vi "demo2.vi"() -> (0 "Error Out":errorcluster)   [LabVIEW 2024]
uses:
  Alarming-Actor/Source/Alarming Actor/Alarming Actor/Alarming Actor.lvclass
  Alarming-Actor/Source/Alarming Actor UI/Alarming Actor UI.lvclass
  Source/Alarming Strategy/Alarming Actor Strategy.lvclass
  Source/Interfaces/IRead Temperature/IRead Temperature.lvclass
  Source/Interfaces/IWrite Duty Cycle/IWrite Duty Cycle.lvclass
  Source/Interfaces/IReadPressure/IRead Pressure.lvclass
  Source/Interfaces/IRead Dew Point/IRead Dew Point.lvclass
  Source/Interfaces/IRead Humidity/IRead Humidity.lvclass
  Source/Interfaces/IRead H2O Concentration/IRead H2O Concentration.lvclass
  Source/Interfaces/IVirtual Instrument/IVirtual Instrument.lvclass
  Source/Instrument Manager/Instrument Manager.lvclass
  Source/Interfaces/IRunnable/IRunnable.lvclass
  Alarming-Actor/Source/Alarming Actor/Alarming Actor/Alarming Level.ctl
  Supply Control States.ctl
  fd6abf06-3d04-4345-ac09-30423c28f45e.vi
  f97e5bf6-71f0-418f-9a98-3962d6491cca.vi
  a312cea4-3cc5-4a6b-8bfd-08d3799cec9d.vi
  458dd3b6-fbb4-4b61-9531-a4b22eeaadbe.vi
  96793fb8-29df-4936-a506-fddfdbc4ff2a.vi
  Progress Bar Switch.ctl
  Stack.ctl
panel:
  out "Stack2":T1 {"Power-Setpoint" format="%d %"; "Purge Valve" scale=0.0..100.0; "Supply Valve" scale=0.0..100.0; "Switch" scale=0.0..100.0; "Voltage" format="%#.2f V"; "Current" format="%#.2f A"; "Pressure" format="%#.0f mbar"; "Thermometer" format="%#.1f °C"; "Fan" format="%d %"; "Power" format="%d W"}
  out "Stack1":T1 {"Power-Setpoint" format="%d %"; "Purge Valve" scale=0.0..100.0; "Supply Valve" scale=0.0..100.0; "Switch" scale=0.0..100.0; "Voltage" format="%#.2f V"; "Current" format="%#.2f A"; "Pressure" format="%#.0f mbar"; "Thermometer" format="%#.1f °C"; "Fan" format="%d %"; "Power" format="%d W"}
  out "Stack Temps":T3(graph) caption="Stack Temperatures °C"
  out "Stack Temperatures":T4(graph)
  in  "Stop Button":bool
  in  "Start Button":bool
  in  "Shutdown Button":bool
  out "Identifier":string
  out "Alarming Level":T5
  out "Temperature":dbl format="%.2f °C"
  out "Time Stamp t":timestamp format="%<%x %.3X>T"
  out "Pressure":dbl format="%d mbar a"
  out "Time Stamp p":timestamp format="%<%x %.3X>T"
  out "Dew Point":dbl format="%.2f °C"
  out "Time Stamp d":timestamp format="%<%x %.3X>T"
  out "Absolute Humidity":dbl format="%.1f g/m³"
  out "Time Stamp h":timestamp format="%<%x %.3X>T"
  out "H2O Concentration":dbl format="%d Vol.-%"
  out "Time Stamp c":timestamp format="%<%x %.3X>T"
  out "Main Supply":T6(graph)
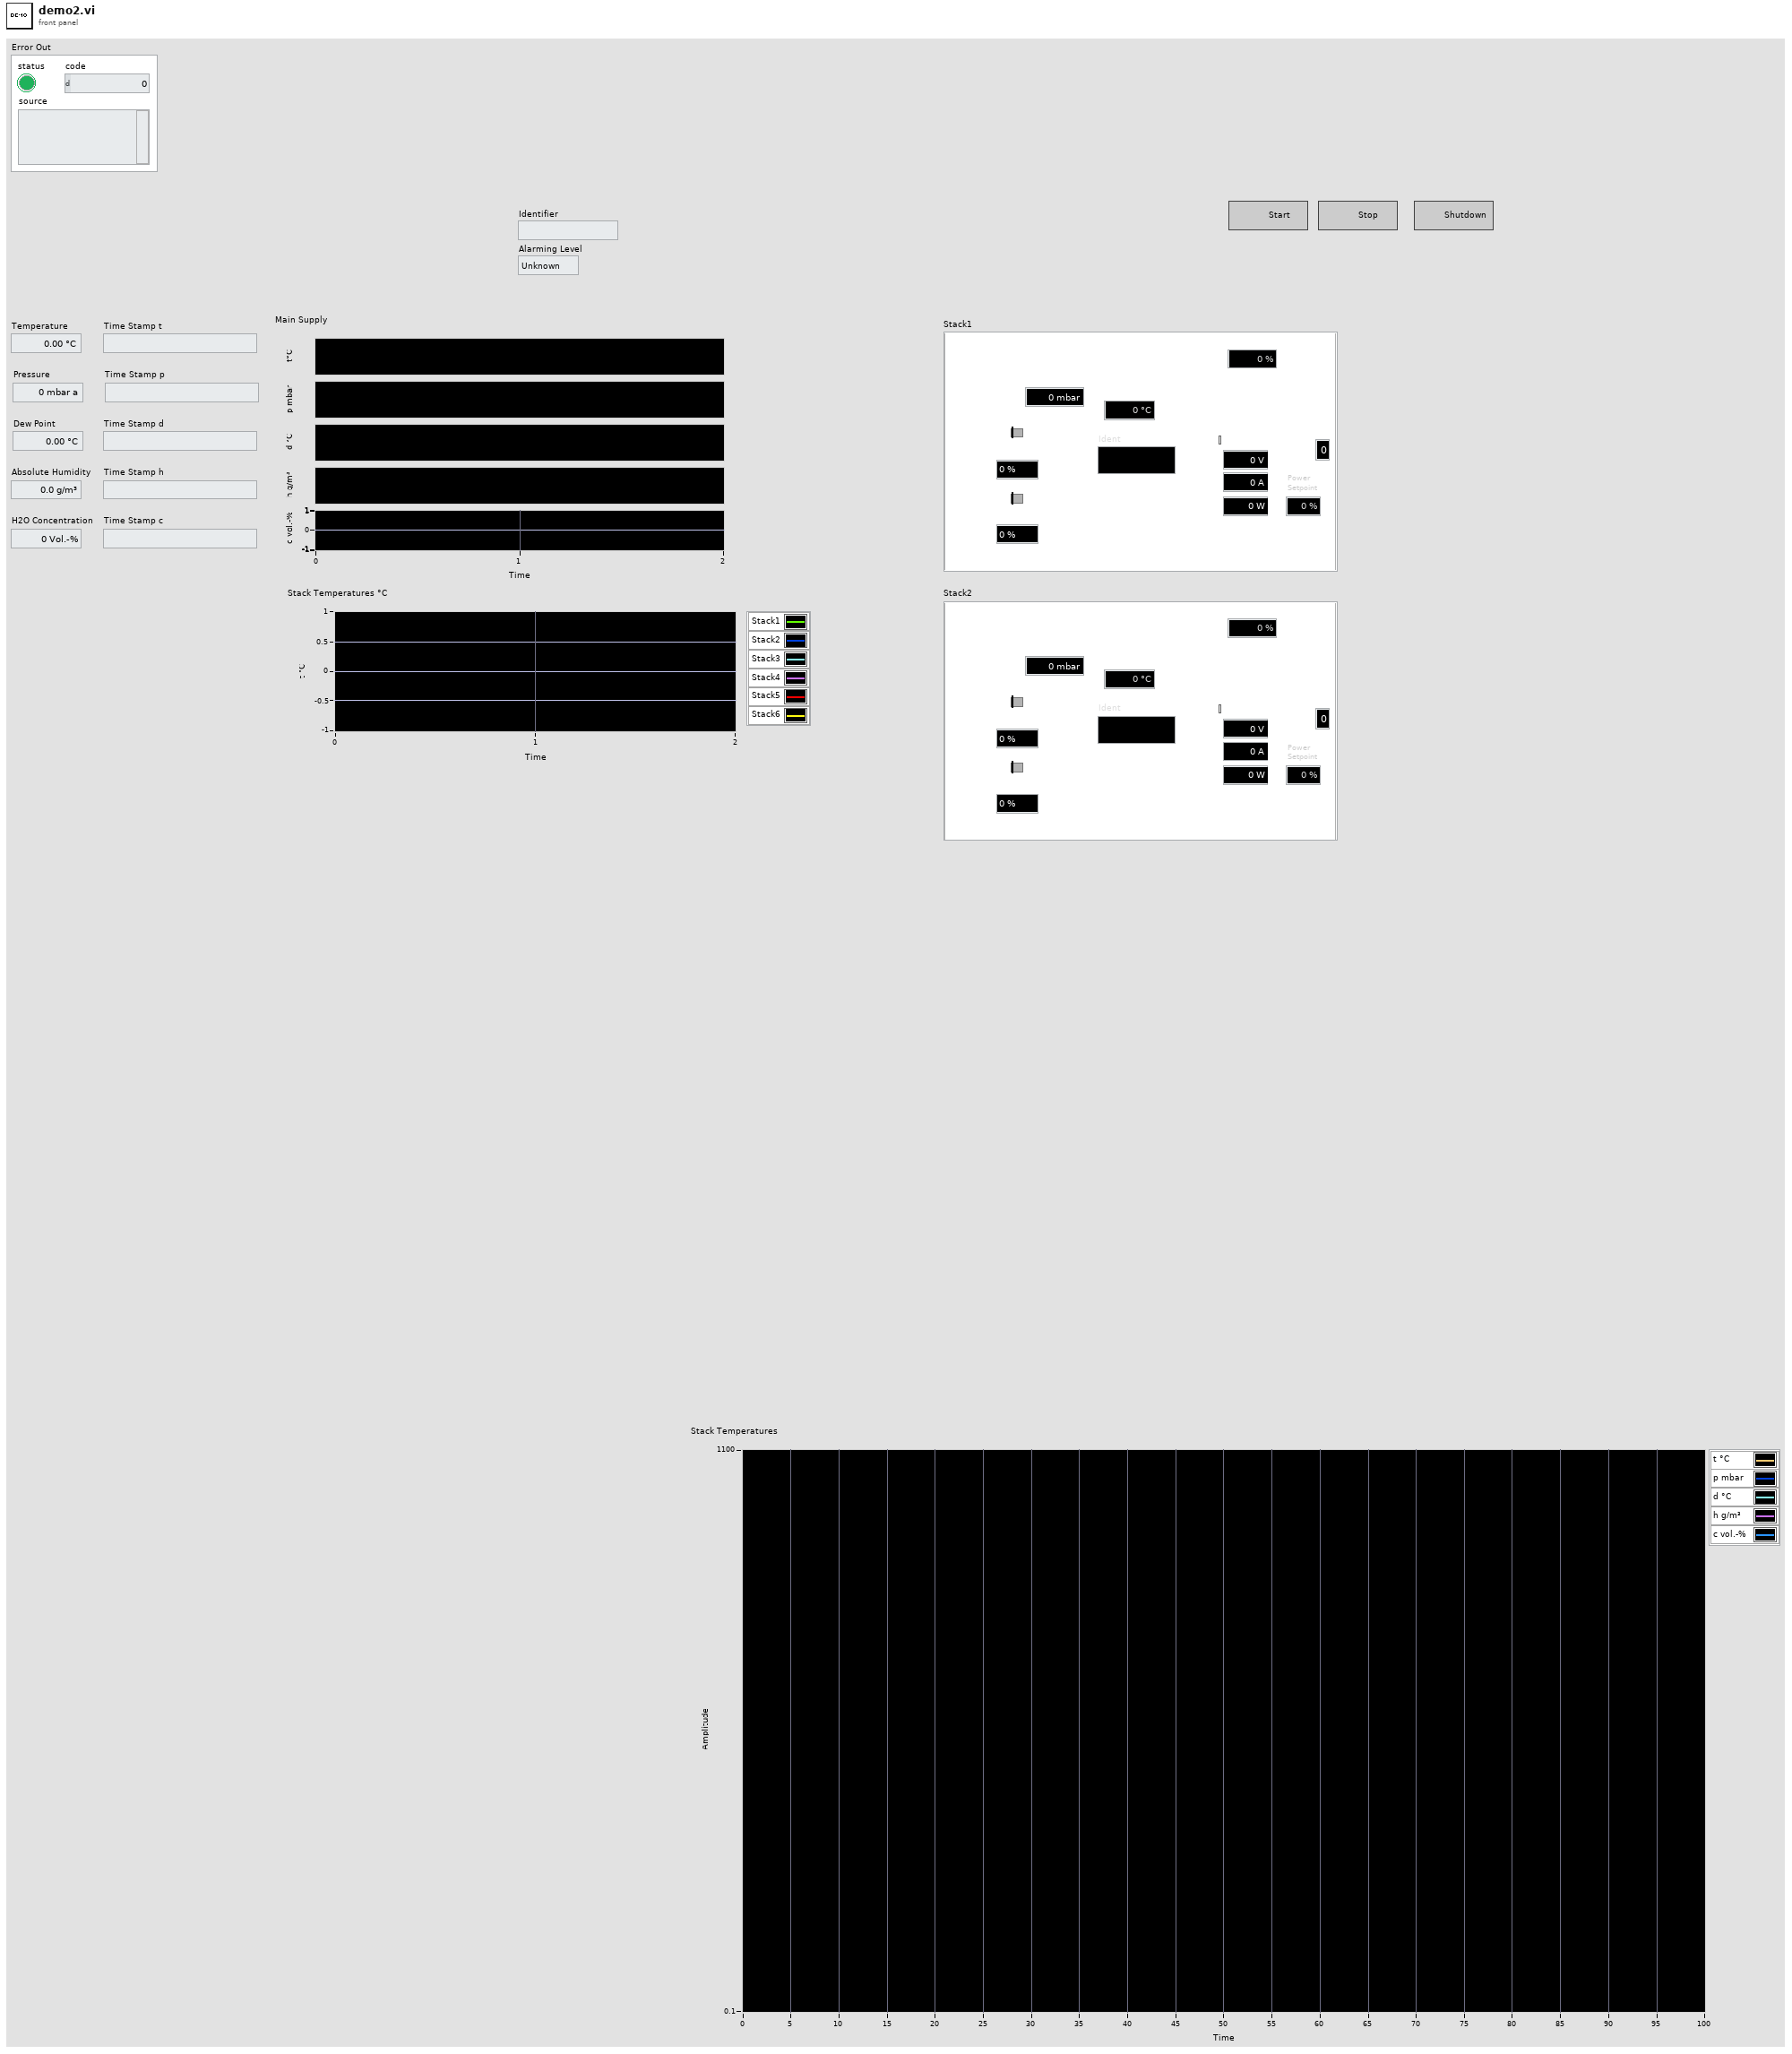
[diagram p1: front panel]
types:
  T1 = typedef "Stack.ctl" = cluster{"Ident":string, "Power":dbl, "Fan":dbl, "Thermometer":dbl, "MCU":u8, "Pressure":dbl, "Current":dbl, "Voltage":dbl, "Switch 2":bool, "Switch 3":bool, "Switch":T2, "Switch 4":bool, "Supply Valve":dbl, "Purge Valve":dbl, "Power-Setpoint":dbl}
  T2 = typedef "Progress Bar Switch.ctl" = u8
  T3 = cluster{"[0]":dbl, "[1]":dbl, "[2]":dbl, "[3]":dbl, "[4]":dbl, "[5]":dbl}
  T4 = cluster{"Temperature":dbl, "Temperature":dbl, "Temperature":dbl, "Temperature":dbl, "Temperature":dbl, "Temperature":dbl}
  T5 = typedef "Alarming Actor.lvlib/Alarming Actor.lvclass/Alarming Level.ctl" = enum16{"Unknown", "OK", "Warning", "Critical"}
  T6 = cluster{"Temperature":dbl, "Pressure":dbl, "Dew Point":dbl, "Humidity":dbl, "H2O Concentration":dbl}
  T7 = typedef "Supply Control States.ctl" = enum16{"Idle", "Run", "Shutdown"}
  T8 = cluster{"Identifier":string, "Alarming Level":T5}
  T9 = cluster{"Alarm Status Changed":refnum<user-event>}
  T10 = typedef "Rendezvous RefNum" = refnum<k1>
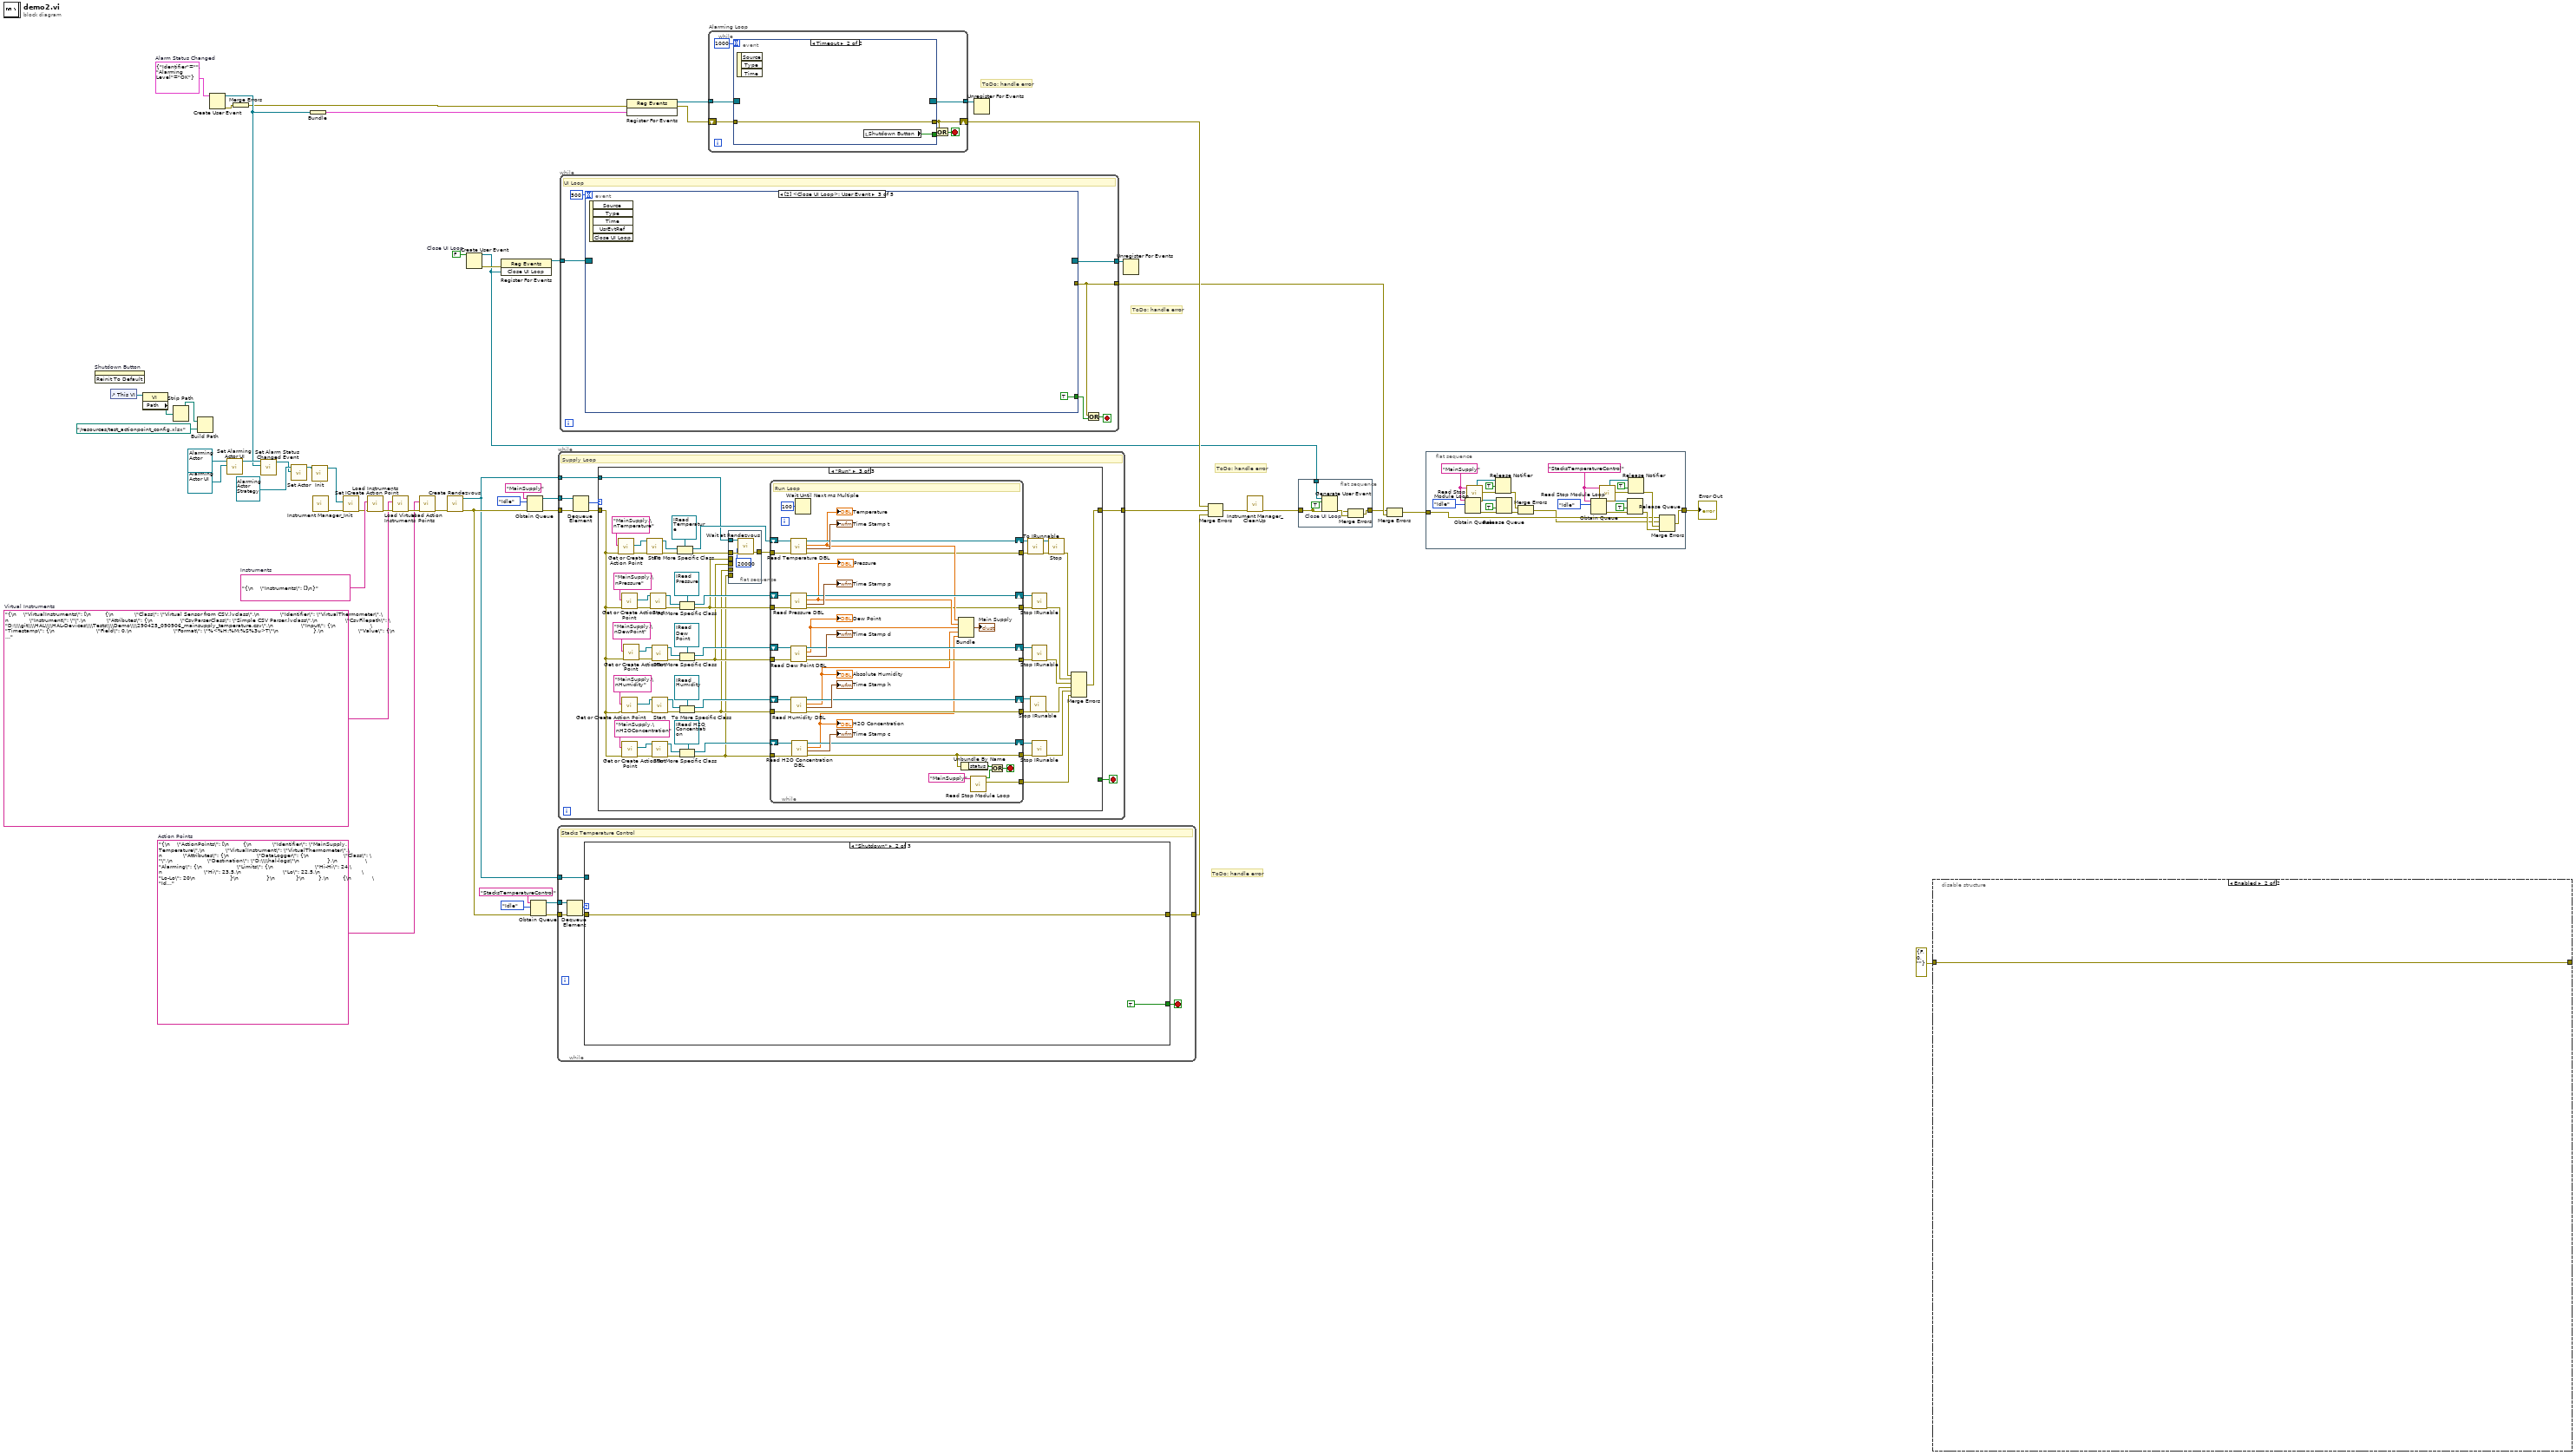
[diagram p0: block diagram]
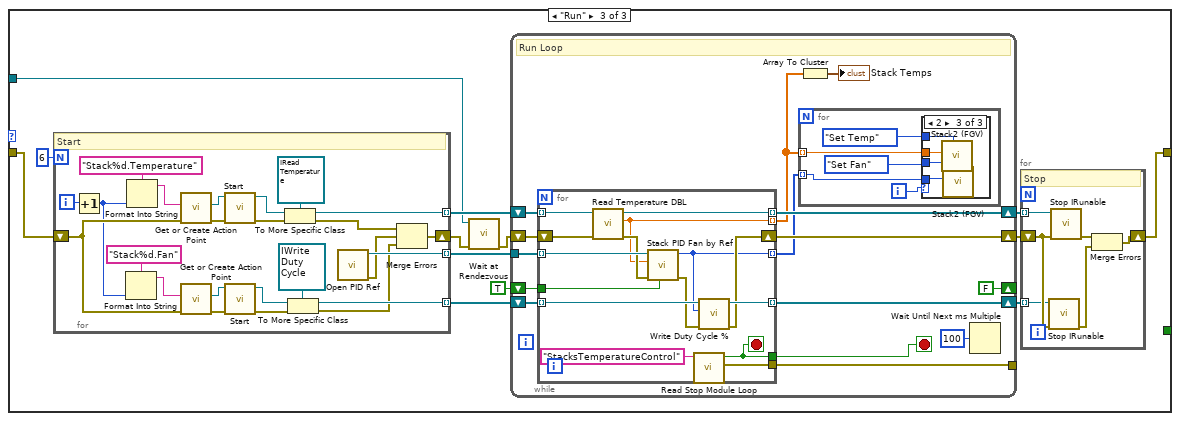
[diagram p3: hidden frame]
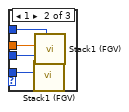
[diagram p5: hidden frame]
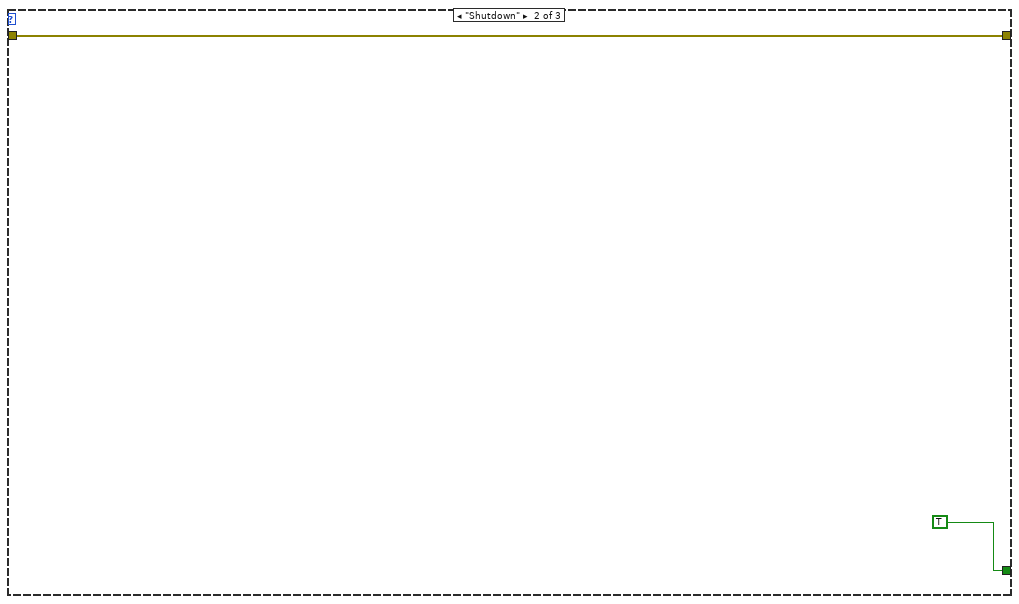
[diagram p7: hidden frame]
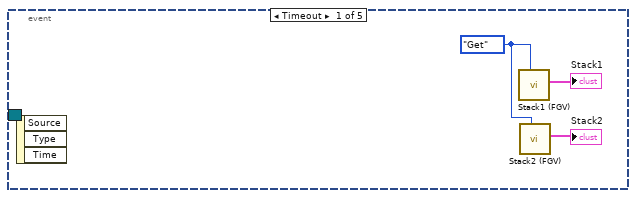
[diagram p8: hidden frame]
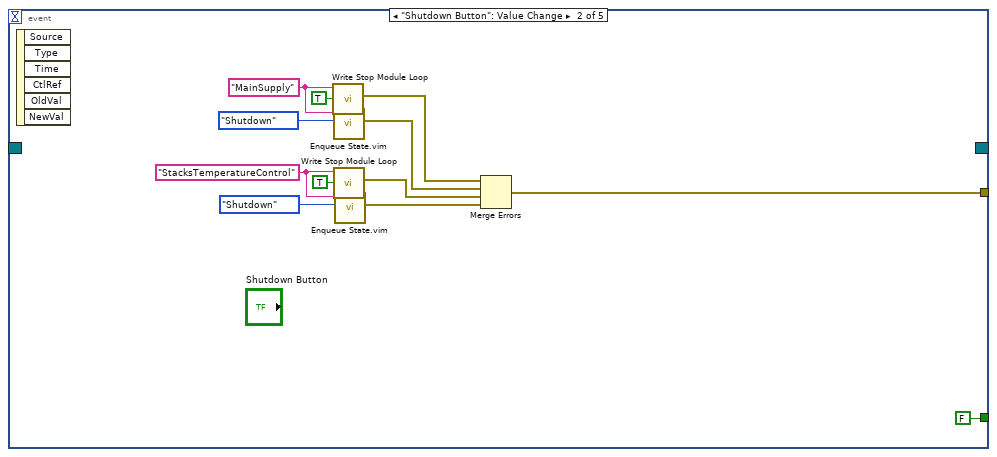
[diagram p9: hidden frame]
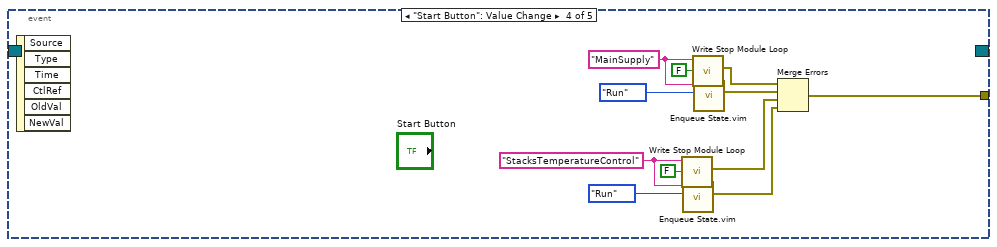
[diagram p10: hidden frame]
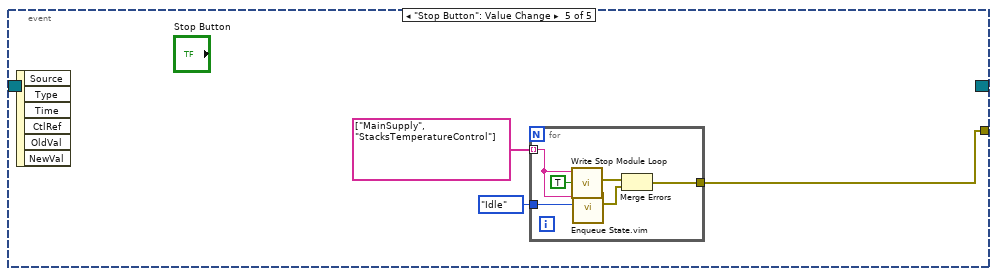
[diagram p11: hidden frame]
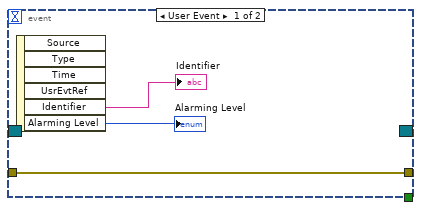
[diagram p12: hidden frame]
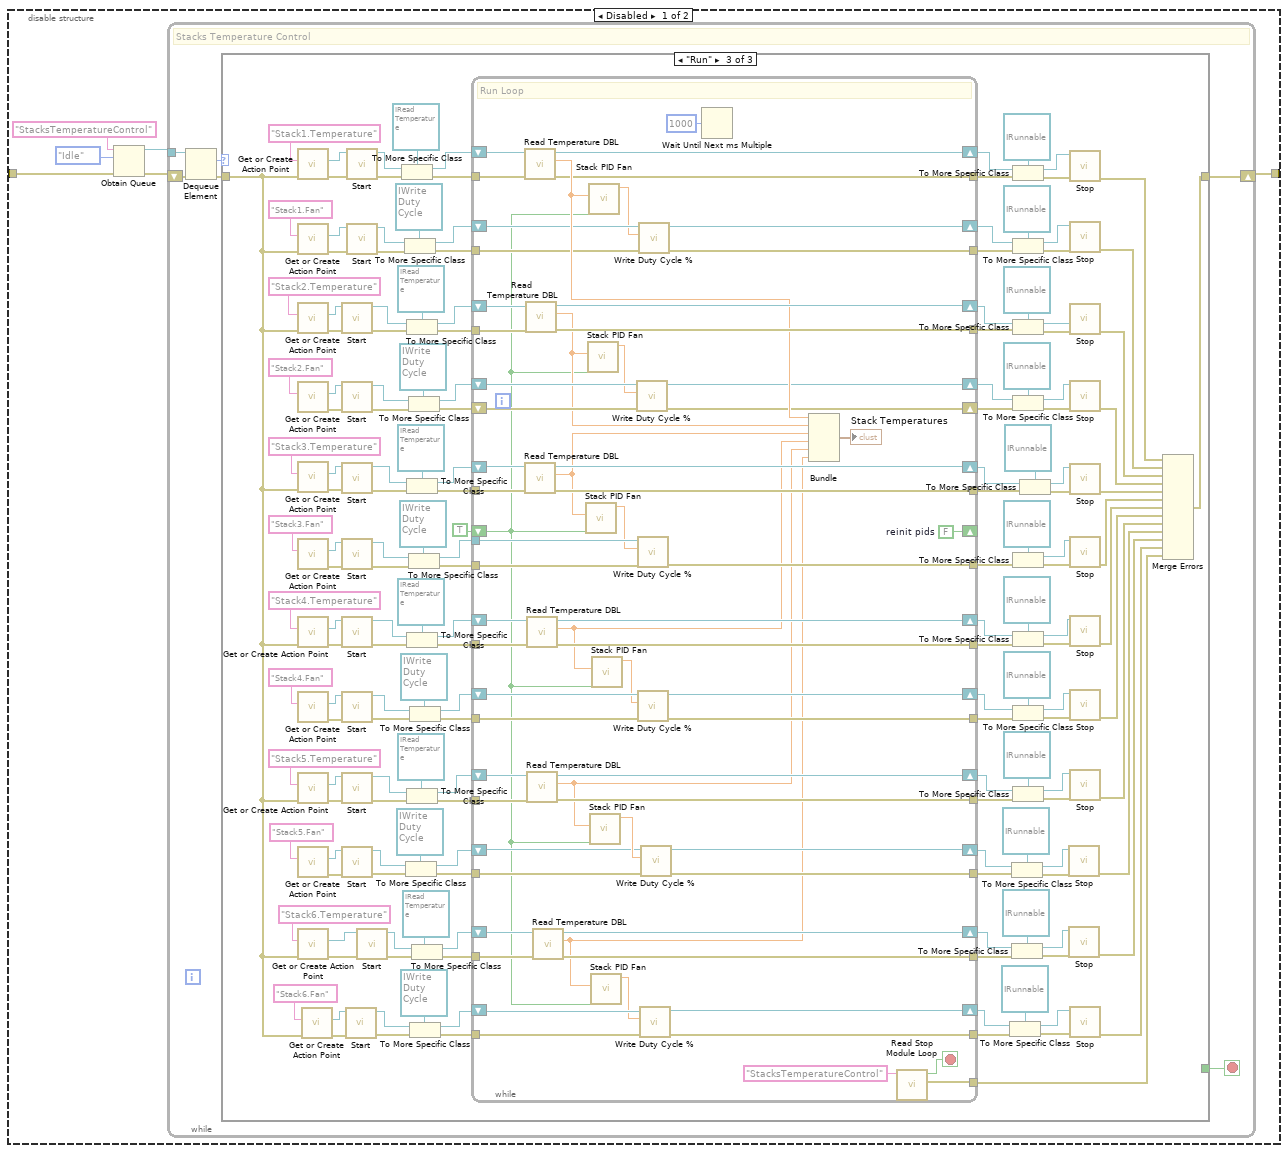
[diagram p13: hidden frame]
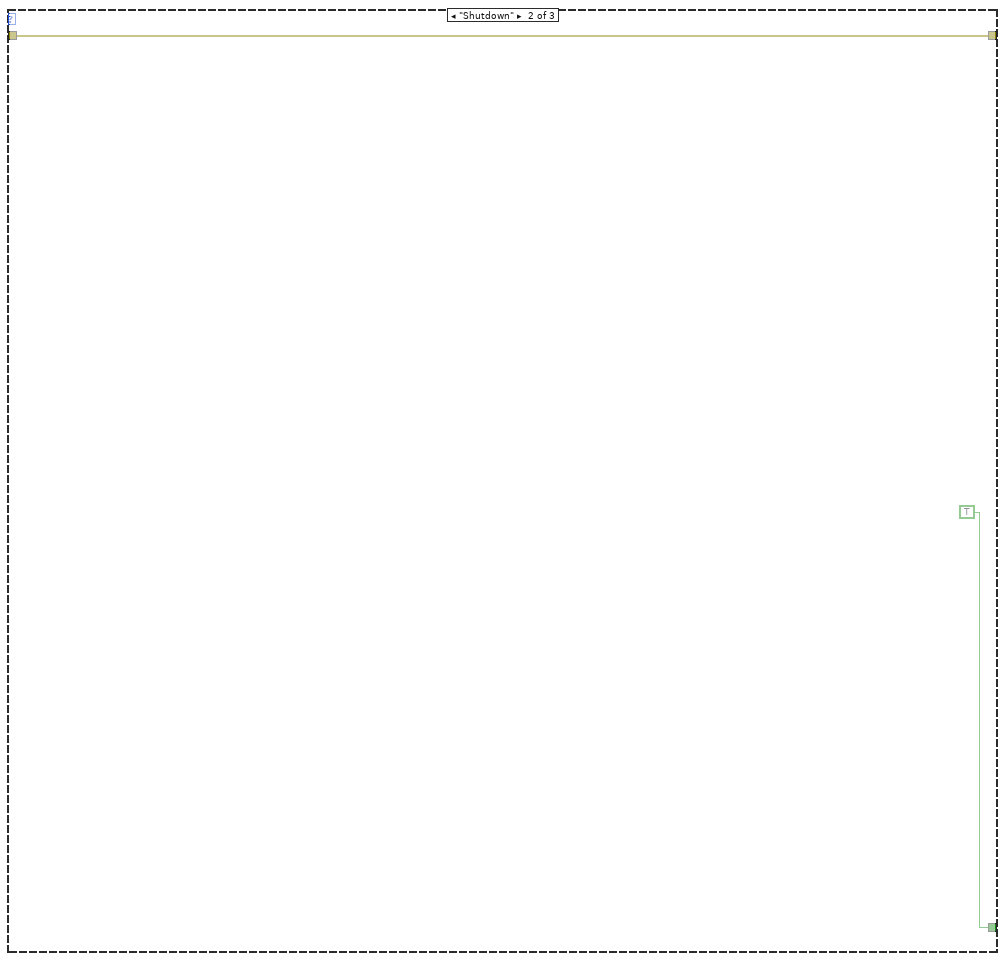
[diagram p15: hidden frame]
diagram:
  w22 = FALSE  # Close UI Loop
  w34 = "{\n    \"VirtualInstruments\": [\n        {\n            \"Class\": \"Virtual Sensor from CSV.lvclass\",\n            \"Identifier\": \"VirtualThermometer\",\n            \"Instrument\": \"\",\n            \"Attributes\": {\n                \"CsvParserClass\": \"Simple CSV Parser.lvclass\",\n                \"CsvFilepath\": \"D:\\\\git\\\\HAL\\\\HAL-Devices\\\\Tests\\\\Demo\\\\290425_090906_mainsupply_temperature.csv\",\n                \"Input\": {\n                    \"Timestamp\": {\n                        \"Field\": 0,\n                        \"Format\": \"%<%H:%M:%S%3u>T\"\n                    },\n                    \"Value\": {\n                        \"Field\": 1\n                    }\n                },\n                \"Seperator\": \",\"\n            }\n        },\n        {\n            \"Class\": \"Virtual Sensor from CSV.lvclass\",\n            \"Identifier\": \"VirtualPressureSensor\",\n            \"Instrument\": \"\",\n            \"Attributes\": {\n                \"CsvParserClass\": \"Simple CSV Parser.lvclass\",\n                \"CsvFilepath\": \"D:\\\\git\\\\HAL\\\\HAL-Devices\\\\Tests\\\\Demo\\\\290425_090906_mainsupply_pressure.csv\",\n                \"Input\": {\n                    \"Timestamp\": {\n                        \"Field\": 0,\n                        \"Format\": \"%<%H:%M:%S%3u>T\"\n                    },\n                    \"Value\": {\n                        \"Field\": 1\n                    }\n                },\n                \"Seperator\": \",\"\n            }\n        },\n        {\n            \"Class\": \"Virtual Sensor from CSV.lvclass\",\n            \"Identifier\": \"VirtualDewPointSensor\",\n            \"Instrument\": \"\",\n            \"Attributes\": {\n                \"CsvParserClass\": \"Simple CSV Parser.lvclass\",\n                \"CsvFilepath\": \"D:\\\\git\\\\HAL\\\\HAL-Devices\\\\Tests\\\\Demo\\\\290425_090906_mainsupply_dewpoint.csv\",\n                \"Input\": {\n                    \"Timestamp\": {\n                        \"Field\": 0,\n                        \"Format\": \"%<%H:%M:%S%3u>T\"\n                    },\n                    \"Value\": {\n                        \"Field\": 1\n                    }\n                },\n                \"Seperator\": \",\"\n            }\n        },\n        {\n            \"Class\": \"Virtual Sensor from CSV.lvclass\",\n            \"Identifier\": \"VirtualHumiditySensor\",\n            \"Instrument\": \"\",\n            \"Attributes\": {\n                \"CsvParserClass\": \"Simple CSV Parser.lvclass\",\n                \"CsvFilepath\": \"D:\\\\git\\\\HAL\\\\HAL-Devices\\\\Tests\\\\Demo\\\\290425_090906_mainsupply_humidity.csv\",\n                \"Input\": {\n                    \"Timestamp\": {\n                        \"Field\": 0,\n                        \"Format\": \"%<%H:%M:%S%3u>T\"\n                    },\n                    \"Value\": {\n                        \"Field\": 1\n                    }\n                },\n                \"Seperator\": \",\"\n            }\n        },\n        {\n            \"Class\": \"Virtual Sensor from CSV.lvclass\",\n            \"Identifier\": \"VirtualH2OConcentrationSensor\",\n            \"Instrument\": \"\",\n            \"Attributes\": {\n                \"CsvParserClass\": \"Simple CSV Parser.lvclass\",\n                \"CsvFilepath\": \"D:\\\\git\\\\HAL\\\\HAL-Devices\\\\Tests\\\\Demo\\\\290425_090906_mainsupply_h2oconcentration.csv\",\n                \"Input\": {\n                    \"Timestamp\": {\n                        \"Field\": 0,\n                        \"Format\": \"%<%H:%M:%S%3u>T\"\n                    },\n                    \"Value\": {\n                        \"Field\": 1\n                    }\n                },\n                \"Seperator\": \",\"\n            }\n        },\n        {\n            \"Class\": \"Virtual Sensor from CSV.lvclass\",\n            \"Identifier\": \"act_T_Stack_1_out_Th\",\n            \"Instrument\": \"\",\n            \"Attributes\": {\n                \"CsvParserClass\": \"Named Fields Parser.lvclass\",\n                \"CsvFilepath\": \"D:\\\\git\\\\HAL\\\\HAL-Devices\\\\Tests\\\\resources\\\\2024-11-27-17-48-50_Imponator_Last Hope.csv\",\n                \"Input\": {\n                    \"Timestamp\": {\n                        \"Field\": \"Time in sec\",\n                        \"Format\": \"%t\"\n                    },\n                    \"Value\": {\n                        \"Field\": \"act_T_Stack_1_out_Th\"\n                    }\n                },\n                \"Seperator\": \";\"\n            }\n        },\n        {\n            \"Class\": \"Virtual Sensor from CSV.lvclass\",\n            \"Identifier\": \"act_T_Stack_2_out_Th\",\n            \"Instrument\": \"\",\n            \"Attributes\": {\n                \"CsvParserClass\": \"Named Fields Parser.lvclass\",\n                \"CsvFilepath\": \"D:\\\\git\\\\HAL\\\\HAL-Devices\\\\Tests\\\\resources\\\\2024-11-27-17-48-50_Imponator_Last Hope.csv\",\n                \"Input\": {\n                    \"Timestamp\": {\n                        \"Field\": \"Time in sec\",\n                        \"Format\": \"%t\"\n                    },\n                    \"Value\": {\n                        \"Field\": \"act_T_Stack_2_out_Th\"\n                    }\n                },\n                \"Seperator\": \";\"\n            }\n        },\n        {\n            \"Class\": \"Virtual Sensor from CSV.lvclass\",\n            \"Identifier\": \"act_T_Stack_3_out_Th\",\n            \"Instrument\": \"\",\n            \"Attributes\": {\n                \"CsvParserClass\": \"Named Fields Parser.lvclass\",\n                \"CsvFilepath\": \"D:\\\\git\\\\HAL\\\\HAL-Devices\\\\Tests\\\\resources\\\\2024-11-27-17-48-50_Imponator_Last Hope.csv\",\n                \"Input\": {\n                    \"Timestamp\": {\n                        \"Field\": \"Time in sec\",\n                        \"Format\": \"%t\"\n                    },\n                    \"Value\": {\n                        \"Field\": \"act_T_Stack_3_out_Th\"\n                    }\n                },\n                \"Seperator\": \";\"\n            }\n        },\n        {\n            \"Class\": \"Virtual Sensor from CSV.lvclass\",\n            \"Identifier\": \"act_T_Stack_4_out_Th\",\n            \"Instrument\": \"\",\n            \"Attributes\": {\n                \"CsvParserClass\": \"Named Fields Parser.lvclass\",\n                \"CsvFilepath\": \"D:\\\\git\\\\HAL\\\\HAL-Devices\\\\Tests\\\\resources\\\\2024-11-27-17-48-50_Imponator_Last Hope.csv\",\n                \"Input\": {\n                    \"Timestamp\": {\n                        \"Field\": \"Time in sec\",\n                        \"Format\": \"%t\"\n                    },\n                    \"Value\": {\n                        \"Field\": \"act_T_Stack_4_out_Th\"\n                    }\n                },\n                \"Seperator\": \";\"\n            }\n        },\n        {\n            \"Class\": \"Virtual Sensor from CSV.lvclass\",\n            \"Identifier\": \"act_T_Stack_5_out_Th\",\n            \"Instrument\": \"\",\n            \"Attributes\": {\n                \"CsvParserClass\": \"Named Fields Parser.lvclass\",\n                \"CsvFilepath\": \"D:\\\\git\\\\HAL\\\\HAL-Devices\\\\Tests\\\\resources\\\\2024-11-27-17-48-50_Imponator_Last Hope.csv\",\n                \"Input\": {\n                    \"Timestamp\": {\n                        \"Field\": \"Time in sec\",\n                        \"Format\": \"%t\"\n                    },\n                    \"Value\": {\n                        \"Field\": \"act_T_Stack_5_out_Th\"\n                    }\n                },\n                \"Seperator\": \";\"\n            }\n        },\n        {\n            \"Class\": \"Virtual Sensor from CSV.lvclass\",\n            \"Identifier\": \"act_T_Stack_6_out_Th\",\n            \"Instrument\": \"\",\n            \"Attributes\": {\n                \"CsvParserClass\": \"Named Fields Parser.lvclass\",\n                \"CsvFilepath\": \"D:\\\\git\\\\HAL\\\\HAL-Devices\\\\Tests\\\\resources\\\\2024-11-27-17-48-50_Imponator_Last Hope.csv\",\n                \"Input\": {\n                    \"Timestamp\": {\n                        \"Field\": \"Time in sec\",\n                        \"Format\": \"%t\"\n                    },\n                    \"Value\": {\n                        \"Field\": \"act_T_Stack_6_out_Th\"\n                    }\n                },\n                \"Seperator\": \";\"\n            }\n        },\n        {\n            \"Class\": \"Virtual PWM Generator.lvclass\",\n            \"Identifier\": \"Virtual PWM Generator\",\n            \"Instrument\": \"\",\n            \"Attributes\": {}\n        }\n    ]\n}"  # Virtual Instruments
  w35 = "{\n    \"Instruments\": []\n}"  # Instruments
  w40 = T8 {"Identifier"="", "Alarming Level"=enum."OK"}  # Alarm Status Changed
  w44 = "{\n    \"ActionPoints\": [\n        {\n            \"Identifier\": \"MainSupply.Temperature\",\n            \"VirtualInstrument\": \"VirtualThermometer\",\n            \"Attributes\": {\n                \"DataLogger\": {\n                    \"Class\": \"\",\n                    \"Destination\": \"D:\\\\hal-logs\"\n                },\n                \"Alarming\": {\n                    \"Limits\": {\n                        \"Hi-Hi\": 24,\n                        \"Hi\": 23.5,\n                        \"Lo\": 22.5,\n                        \"Lo-Lo\": 20\n                    }\n                }\n            }\n        },\n        {\n            \"Identifier\": \"MainSupply.Pressure\",\n            \"VirtualInstrument\": \"VirtualPressureSensor\",\n            \"Attributes\": {\n                \"DataLogger\": {\n                    \"Class\": \"\",\n                    \"Destination\": \"D:\\\\hal-logs\"\n                },\n                \"Alarming\": {\n                    \"Limits\": {\n                        \"Hi-Hi\": 1021,\n                        \"Hi\": 1019,\n                        \"Lo\": 0,\n                        \"Lo-Lo\": 0\n                    }\n                }\n            }\n        },\n        {\n            \"Identifier\": \"MainSupply.DewPoint\",\n            \"VirtualInstrument\": \"VirtualDewPointSensor\",\n            \"Attributes\": {\n                \"DataLogger\": {\n                    \"Class\": \"\",\n                    \"Destination\": \"D:\\\\hal-logs\"\n                },\n                \"Alarming\": {\n                    \"Limits\": {\n                        \"Hi-Hi\": 9,\n                        \"Hi\": 7.5,\n                        \"Lo\": 7,\n                        \"Lo-Lo\": 5\n                    }\n                }\n            }\n        },\n        {\n            \"Identifier\": \"MainSupply.Humidity\",\n            \"VirtualInstrument\": \"VirtualHumiditySensor\",\n            \"Attributes\": {\n                \"DataLogger\": {\n                    \"Class\": \"\",\n                    \"Destination\": \"D:\\\\hal-logs\"\n                },\n                \"Alarming\": {\n                    \"Limits\": {\n                        \"Hi-Hi\": 10,\n                        \"Hi\": 8,\n                        \"Lo\": 6,\n                        \"Lo-Lo\": 4\n                    }\n                }\n            }\n        },\n        {\n            \"Identifier\": \"MainSupply.H2OConcentration\",\n            \"VirtualInstrument\": \"VirtualH2OConcentrationSensor\",\n            \"Attributes\": {\n                \"DataLogger\": {\n                    \"Class\": \"\",\n                    \"Destination\": \"D:\\\\hal-logs\"\n                },\n                \"Alarming\": {\n                    \"Limits\": {\n                        \"Hi-Hi\": 3,\n                        \"Hi\": 2,\n                        \"Lo\": 0,\n                        \"Lo-Lo\": 0\n                    }\n                }\n            }\n        },\n        {\n            \"Identifier\": \"Stack1.Temperature\",\n            \"VirtualInstrument\": \"act_T_Stack_1_out_Th\",\n            \"Attributes\": {\n                \"DataLogger\": {\n                    \"Class\": \"\",\n                    \"Destination\": \"D:\\\\hal-logs\"\n                },\n                \"Alarming\": {\n                    \"Limits\": {\n                        \"Hi-Hi\": 50,\n                        \"Hi\": 45,\n                        \"Lo\": 0,\n                        \"Lo-Lo\": 0\n                    }\n                }\n            }\n        },\n        {\n            \"Identifier\": \"Stack2.Temperature\",\n            \"VirtualInstrument\": \"act_T_Stack_2_out_Th\",\n            \"Attributes\": {\n                \"DataLogger\": {\n                    \"Class\": \"\",\n                    \"Destination\": \"D:\\\\hal-logs\"\n                },\n                \"Alarming\": {\n                    \"Limits\": {\n                        \"Hi-Hi\": 50,\n                        \"Hi\": 45,\n                        \"Lo\": 0,\n                        \"Lo-Lo\": 0\n                    }\n                }\n            }\n        },\n        {\n            \"Identifier\": \"Stack3.Temperature\",\n            \"VirtualInstrument\": \"act_T_Stack_3_out_Th\",\n            \"Attributes\": {\n                \"DataLogger\": {\n                    \"Class\": \"\",\n                    \"Destination\": \"D:\\\\hal-logs\"\n                },\n                \"Alarming\": {\n                    \"Limits\": {\n                        \"Hi-Hi\": 50,\n                        \"Hi\": 45,\n                        \"Lo\": 0,\n                        \"Lo-Lo\": 0\n                    }\n                }\n            }\n        },\n        {\n            \"Identifier\": \"Stack4.Temperature\",\n            \"VirtualInstrument\": \"act_T_Stack_4_out_Th\",\n            \"Attributes\": {\n                \"DataLogger\": {\n                    \"Class\": \"\",\n                    \"Destination\": \"D:\\\\hal-logs\"\n                },\n                \"Alarming\": {\n                    \"Limits\": {\n                        \"Hi-Hi\": 50,\n                        \"Hi\": 45,\n                        \"Lo\": 0,\n                        \"Lo-Lo\": 0\n                    }\n                }\n            }\n        },\n        {\n            \"Identifier\": \"Stack5.Temperature\",\n            \"VirtualInstrument\": \"act_T_Stack_5_out_Th\",\n            \"Attributes\": {\n                \"DataLogger\": {\n                    \"Class\": \"\",\n                    \"Destination\": \"D:\\\\hal-logs\"\n                },\n                \"Alarming\": {\n                    \"Limits\": {\n                        \"Hi-Hi\": 50,\n                        \"Hi\": 45,\n                        \"Lo\": 0,\n                        \"Lo-Lo\": 0\n                    }\n                }\n            }\n        },\n        {\n            \"Identifier\": \"Stack6.Temperature\",\n            \"VirtualInstrument\": \"act_T_Stack_6_out_Th\",\n            \"Attributes\": {\n                \"DataLogger\": {\n                    \"Class\": \"\",\n                    \"Destination\": \"D:\\\\hal-logs\"\n                },\n                \"Alarming\": {\n                    \"Limits\": {\n                        \"Hi-Hi\": 50,\n                        \"Hi\": 45,\n                        \"Lo\": 0,\n                        \"Lo-Lo\": 0\n                    }\n                }\n            }\n        },\n        {\n            \"Identifier\": [\n                \"Stack1.Fan\",\n                \"Stack2.Fan\",\n                \"Stack3.Fan\",\n                \"Stack4.Fan\",\n                \"Stack5.Fan\",\n                \"Stack6.Fan\"\n            ],\n            \"VirtualInstrument\": \"Virtual PWM Generator\",\n            \"Attributes\": {\n                \"DataLogger\": {\n                    \"Class\": \"\",\n                    \"Destination\": \"D:\\\\hal-logs\"\n                },\n                \"Alarming\": {\n                    \"Limits\": {\n                        \"Hi-Hi\": 101,\n                        \"Hi\": 100,\n                        \"Lo\": 14,\n                        \"Lo-Lo\": 0\n                    }\n                }\n            }\n        }\n    ]\n}"  # Action Points
  # "ToDo: handle error"
  # "ToDo: handle error"
  # "ToDo: handle error"
  # "ToDo: handle error"
  n1 = invoke on="Shutdown Button" class="Bool (strict)" method="Reinit To Default"() -> ()  [unwired: 3 in, 3 out]
  n2 = control-ref of="This VI"() -> (w48:refnum<vi>)
  n3 = property class="VI"(reference=w48) -> ("Path"=w47:path)  [unwired: 1 in, 2 out]
  n4 = Strip Path(path=w47) -> (stripped path=w45:path)  [unwired: 1 out]
  n5 = Build Path(base path=w45, name or relative path=path "../resources/test_actionpoint_config.xlsx") -> ()  [unwired: 1 out]
  n6 = Create User Event(user event datatype=w40) -> (user event=w37:refnum<user-event>, error out=w16:errorcluster)  [unwired: 1 in]
  n7 = call "Set Alarming Actor UI.vi"("UI Actor"=refnum<class "Alarming Actor UI.lvclass"> refnum ("Alarming Actor UI.lvlib:Alarming Actor UI.lvclass"), "Alarming Actor in"=refnum<class "Alarming Actor.lvclass"> refnum ("Alarming Actor.lvlib:Alarming Actor.lvclass")) -> ("Alarming Actor out"=w42:refnum<class "Alarming Actor.lvclass">)  [unwired: 9 in]
  n8 = Merge Errors(w16) -> (w17:errorcluster)
  n9 = call "Set Alarm Status Changed Event.vi"("Alarm Status Changed"=w37, "Alarming Actor in"=w42) -> ("Alarming Actor out"=w4:refnum<class "Alarming Actor.lvclass">)  [unwired: 9 in]
  n10 = call-dynamic "Set Actor.vi"("Actor"=w4, "Alarming Strategy in"=refnum<class "Alarming Actor Strategy.lvclass"> refnum ("Alarming Actor Strategy.lvclass")) -> ("Alarming Strategy out"=w2:refnum<class "Alarming Actor Strategy.lvclass">)  [unwired: 9 in]
  n11 = Bundle("Alarm Status Changed"=w37) -> (w15:T9)  [unwired: 1 in]
  n12 = call-dynamic "Init.vi"("Alarming Strategy in"=w2) -> ("Alarming Strategy out"=w1:refnum<class "Alarming Actor Strategy.lvclass">)  [unwired: 9 in, 1 out]
  n13 = call "Instrument Manager_Init.vi"() -> ("Error Out"=w52:errorcluster)  [unwired: 10 in, 1 out]
  n14 = call "Set ICreate Action Point.vi"("Error In"=w52, "ICreate Action Point"=w1) -> ("Error Out"=w6:errorcluster)  [unwired: 9 in]
  n15 = call "Load Instruments.vi"("Error In"=w6, "Source"=w35) -> ("Error Out"=w51:errorcluster)  [unwired: 9 in]
  n16 = call "Load Virtual Instruments.vi"("Error In"=w51, "Source"=w34) -> ("Error Out"=w49:errorcluster)  [unwired: 9 in]
  n17 = call "Load Action Points.vi"("Error In"=w49, "Source"=w44) -> ("Error Out"=w11:errorcluster)  [unwired: 9 in]
  n18 = call <vilib>:"Create Rendezvous.vi"("error in (no error)"=w11) -> ("error out"=w10:errorcluster, "rendezvous"=w9:T10)  [unwired: 4 in, 1 out]
  n19 = Create User Event(user event datatype=w22) -> (user event=w12:refnum<user-event>, error out=w23:errorcluster)  [unwired: 1 in]
  n20 = register-events(error in=w23, w12) -> (reference out=w24:refnum<event-registration>)  [unwired: 1 in, 1 out]
  n21 = Obtain Queue(name (unnamed)="MainSupply", element data type=Supply_Control_States."Idle" ("Supply Control States"), error in (no error)=w10) -> (queue out=w31:refnum<queue>, error out=w33:errorcluster)  [unwired: 2 in, 1 out]
  n22 = Obtain Queue(name (unnamed)="StacksTemperatureControl", element data type=Supply_Control_States."Idle" ("Supply Control States"), error in (no error)=w10) -> (queue out=w26:refnum<queue>, error out=w27:errorcluster)  [unwired: 2 in, 1 out]
  n23 = while "Supply Loop" {
    tunnel: w26 -> [w54]
    tunnel: w9 -> [w53]
    tunnel: w27 -> [w58]
    tunnel: [w59] -> w20
    stop <- w55 stop-if-true
    # "Stacks Temperature Control"
    n24 = Dequeue Element(queue=w54, error in (no error)=w58) -> (element=w56:T7, error out=w57:errorcluster)  [unwired: 1 in, 2 out]
    n25 = case shown="\"Shutdown\"" w56 {
      tunnel: [w60 w62 w70] -> w59
      tunnel: w57 -> [w60 w62 w66]
      tunnel: [_ TRUE _] -> w55
      tunnel: w53 -> [_ _ w63]
      frame "Idle", Default {
      }
      frame "Shutdown" {
      }
      frame "Run" {
        n26 = for {
          N: 6 -> [_]
          tunnel: [w147] -> w73 mode=indexing
          tunnel: [w136] -> w72 mode=indexing
          shift-right: [w128] -> w65
          shift-left: w66 -> [w135]
          tunnel: [w127] -> w67 mode=indexing
          i -> [w130]
          # "Start"
          n27 = Increment(x=w130) -> (x+1=w129:i32)
          n28 = Format Into String(format string="Stack%d.Fan" ("Action Point Identifier"), w129) -> (resulting string=w132:string)  [unwired: 2 in, 1 out]
          n29 = Format Into String(format string="Stack%d.Temperature" ("Instrument Identifier"), w129) -> (resulting string=w133:string)  [unwired: 2 in, 1 out]
          n30 = call "Get or Create Action Point.vi"("Error In"=w135, "Action Point Identifier"=w133) -> ("Error Out"=w143:errorcluster, "IAction Point"=w142:refnum<class "IVirtual Instrument.lvclass">)  [unwired: 8 in]
          n31 = call "Get or Create Action Point.vi"("Error In"=w135, "Action Point Identifier"=w132) -> ("Error Out"=w137:errorcluster, "IAction Point"=w140:refnum<class "IVirtual Instrument.lvclass">)  [unwired: 8 in]
          n32 = call-dynamic "Start.vi"("error in"=w143, "IRunnable in"=w142) -> ("error out"=w145:errorcluster, "IRunnable out"=w144:refnum<class "IVirtual Instrument.lvclass">)  [unwired: 8 in]
          n33 = call-dynamic "Start.vi"("error in"=w137, "IRunnable in"=w140) -> ("error out"=w139:errorcluster, "IRunnable out"=w138:refnum<class "IVirtual Instrument.lvclass">)  [unwired: 8 in]
          n34 = To More Specific Class(target class=refnum<class "IRead Temperature.lvclass"> refnum ("IRead Temperature.lvclass"), reference=w144, error in=w145) -> (specific class reference=w147:refnum<class "IRead Temperature.lvclass">, error out=w146:errorcluster)
          n35 = To More Specific Class(target class=refnum<class "IWrite Duty Cycle.lvclass"> refnum ("IWrite Duty Cycle.lvclass"), reference=w138, error in=w139) -> (specific class reference=w136:refnum<class "IWrite Duty Cycle.lvclass">, error out=w125:errorcluster)
          n36 = call "Open PID Ref.vi"() -> ("error out"=w126:errorcluster, "VI out"=w127:refnum<vi>)  [unwired: 10 in]
          n37 = Merge Errors(w146, w126, w125) -> (w128:errorcluster)
        }
        n38 = call <vilib>:"Wait at Rendezvous.vi"("error in (no error)"=w65, "rendezvous"=w63) -> ("error out"=w64:errorcluster)  [unwired: 3 in, 2 out]
        n39 = while {
          shift-right: [w79] -> w74
          shift-left: w73 -> [w88]
          tunnel: [w87] -> _
          shift-right: [w85] -> w71
          shift-left: w72 -> [w86]
          shift-right: [FALSE] -> _
          shift-left: TRUE -> [w82]
          shift-right: [w84] -> w75
          shift-left: w64 -> [w89]
          tunnel: w67 -> [w81]
          stop <- w83 stop-if-true
          # "Run Loop"
          n40 = for {
            tunnel: [w116] -> w87
            tunnel: [w112] -> w83
            shift-right: [w111] -> w84
            shift-left: w89 -> [w107]
            tunnel: w88 -> [w117] mode=indexing
            tunnel: [w118] -> w79 mode=indexing
            tunnel: w86 -> [w114] mode=indexing
            tunnel: [w113] -> w85 mode=indexing
            tunnel: w82 -> [w109]
            tunnel: w81 -> [w110] mode=indexing
            tunnel: [w105] -> w76 mode=indexing
            tunnel: [w104] -> w77 mode=indexing
            stop <- w112 stop-if-true
            n41 = call-dynamic "Read Temperature DBL.vi"("error in"=w107, "IRead Temperature in"=w117) -> ("error out"=w108:errorcluster, "Temperature"=w105:dbl, "IRead Temperature out"=w118:refnum<class "IRead Temperature.lvclass">)  [unwired: 6 in, 1 out]
            n42 = call "Stack PID Fan by Ref.vi"("Reinitialize"=w109, "error in"=w108, "Temperature"=w105, "PID Ref"=w110) -> ("error out"=w106:errorcluster, "Output"=w104:u8)  [unwired: 6 in]
            n43 = call "Read Stop Module Loop.vi"("Module Ident"="StacksTemperatureControl" ("name (unnamed)")) -> ("error out"=w116:errorcluster, "Stop"=w112:bool)  [unwired: 8 in, 1 out]
            n44 = call-dynamic "Write Duty Cycle %.vi"("error in"=w106, "Duty Cycle"=w104, "IWrite Duty Cycle in"=w114) -> ("error out"=w111:errorcluster, "IWrite Duty Cycle out"=w113:refnum<class "IWrite Duty Cycle.lvclass">)  [unwired: 7 in]
          }
          n45 = for {
            tunnel: w77 -> [w91] mode=indexing
            tunnel: w76 -> [w94] mode=indexing
            i -> [w95]
            n46 = case shown="2" w95 {
              tunnel: w94 -> [_ w99 w102]
              tunnel: enum16{"Get", "Set Temp", "Set Fan"}."Set Temp" ("Action") -> [_ w98 w103]
              tunnel: enum16{"Get", "Set Temp", "Set Fan"}."Set Fan" ("Action") -> [_ w97 w101]
              tunnel: w91 -> [_ w96 w100]
              frame Default {
              }
              frame 1 {
                n47 = call "Stack1 (FGV).vi"("Action"=w97, "Data Element"=w96) -> ()  [unwired: 9 in, 1 out]
                n48 = call "Stack1 (FGV).vi"("Action"=w98, "Data Element"=w99) -> ()  [unwired: 9 in, 1 out]
              }
              frame 2 {
                n49 = call "Stack2 (FGV).vi"("Action"=w103, "Data Element"=w102) -> ()  [unwired: 9 in, 1 out]
                n50 = call "Stack2 (FGV).vi"("Action"=w101, "Data Element"=w100) -> ()  [unwired: 9 in, 1 out]
              }
            }
          }
          n51 = Array To Cluster(array=w76) -> (cluster=→"Stack Temps":T3)
          n52 = Wait Until Next ms Multiple(millisecond multiple=u32 100) -> ()  [unwired: 1 out]
        }
        n53 = for {
          tunnel: w74 -> [w119] mode=indexing
          tunnel: w71 -> [w120] mode=indexing
          shift-right: [w124] -> w70
          shift-left: w75 -> [w122]
          # "Stop"
          n54 = call "Stop IRunable.vi"("error in"=w122, "IRunnable Object"=w120) -> ("error out"=w121:errorcluster)  [unwired: 8 in, 1 out]
          n55 = call "Stop IRunable.vi"("error in"=w122, "IRunnable Object"=w119) -> ("error out"=w123:errorcluster)  [unwired: 8 in, 1 out]
          n56 = Merge Errors(w123, w121) -> (w124:errorcluster)
        }
      }
    }
  }
  n57 = while "Supply Loop" {
    tunnel: w31 -> [w152]
    tunnel: w9 -> [w149]
    tunnel: w33 -> [w154]
    tunnel: [w155] -> w50
    stop <- w150 stop-if-true
    # "Supply Loop"
    n58 = Dequeue Element(queue=w152, error in (no error)=w154) -> (element=w151:T7, error out=w153:errorcluster)  [unwired: 1 in, 2 out]
    n59 = case shown="\"Run\"" w151 {
      tunnel: [w156 w158 w219] -> w155
      tunnel: w153 -> [w156 w158 w189]
      tunnel: [_ TRUE _] -> w150
      tunnel: w149 -> [_ _ w180]
      frame "Idle", Default {
      }
      frame "Shutdown" {
      }
      frame "Run" {
        n60 = call "Get or Create Action Point.vi"("Error In"=w189, "Action Point Identifier"="MainSupply.\nTemperature" ("Instrument Identifier")) -> ("Error Out"=w207:errorcluster, "IAction Point"=w205:refnum<class "IVirtual Instrument.lvclass">)  [unwired: 8 in]
        n61 = call "Get or Create Action Point.vi"("Error In"=w189, "Action Point Identifier"="MainSupply.\nPressure" ("Virtual Instrument Identifier")) -> ("Error Out"=w204:errorcluster, "IAction Point"=w201:refnum<class "IVirtual Instrument.lvclass">)  [unwired: 8 in]
        n62 = call "Get or Create Action Point.vi"("Error In"=w189, "Action Point Identifier"="MainSupply.\nHumidity" ("Virtual Instrument Identifier")) -> ("Error Out"=w193:errorcluster, "IAction Point"=w190:refnum<class "IVirtual Instrument.lvclass">)  [unwired: 8 in]
        n63 = call "Get or Create Action Point.vi"("Error In"=w189, "Action Point Identifier"="MainSupply.\nH2OConcentration" ("Virtual Instrument Identifier")) -> ("Error Out"=w186:errorcluster, "IAction Point"=w187:refnum<class "IVirtual Instrument.lvclass">)  [unwired: 8 in]
        n64 = call "Get or Create Action Point.vi"("Error In"=w189, "Action Point Identifier"="MainSupply.\nDewPoint" ("Instrument Identifier")) -> ("Error Out"=w198:errorcluster, "IAction Point"=w197:refnum<class "IVirtual Instrument.lvclass">)  [unwired: 8 in]
        n65 = call-dynamic "Start.vi"("error in"=w207, "IRunnable in"=w205) -> ("error out"=w209:errorcluster, "IRunnable out"=w208:refnum<class "IVirtual Instrument.lvclass">)  [unwired: 8 in]
        n66 = call-dynamic "Start.vi"("error in"=w204, "IRunnable in"=w201) -> ("error out"=w203:errorcluster, "IRunnable out"=w202:refnum<class "IVirtual Instrument.lvclass">)  [unwired: 8 in]
        n67 = call-dynamic "Start.vi"("error in"=w198, "IRunnable in"=w197) -> ("error out"=w200:errorcluster, "IRunnable out"=w199:refnum<class "IVirtual Instrument.lvclass">)  [unwired: 8 in]
        n68 = call-dynamic "Start.vi"("error in"=w186, "IRunnable in"=w187) -> ("error out"=w185:errorcluster, "IRunnable out"=w184:refnum<class "IVirtual Instrument.lvclass">)  [unwired: 8 in]
        n69 = call-dynamic "Start.vi"("error in"=w193, "IRunnable in"=w190) -> ("error out"=w192:errorcluster, "IRunnable out"=w191:refnum<class "IVirtual Instrument.lvclass">)  [unwired: 8 in]
        n70 = To More Specific Class(target class=refnum<class "IRead Temperature.lvclass"> refnum ("IRead Temperature.lvclass"), reference=w208, error in=w209) -> (specific class reference=w210:refnum<class "IRead Temperature.lvclass">, error out=w182:errorcluster)
        n71 = To More Specific Class(target class=refnum<class "IRead Pressure.lvclass"> refnum ("IRead Pressure.lvclass"), reference=w202, error in=w203) -> (specific class reference=w216:refnum<class "IRead Pressure.lvclass">, error out=w167:errorcluster)
        n72 = To More Specific Class(target class=refnum<class "IRead Dew Point.lvclass"> refnum ("IRead Dew Point.lvclass"), reference=w199, error in=w200) -> (specific class reference=w217:refnum<class "IRead Dew Point.lvclass">, error out=w166:errorcluster)
        n73 = To More Specific Class(target class=refnum<class "IRead Humidity.lvclass"> refnum ("IRead Humidity.lvclass"), reference=w191, error in=w192) -> (specific class reference=w214:refnum<class "IRead Humidity.lvclass">, error out=w165:errorcluster)
        n74 = To More Specific Class(target class=refnum<class "IRead H2O Concentration.lvclass"> refnum ("IRead H2O Concentration.lvclass"), reference=w184, error in=w185) -> (specific class reference=w213:refnum<class "IRead H2O Concentration.lvclass">, error out=w164:errorcluster)
        n75 = flat-sequence {
          tunnel: w182 -> [w224]
          tunnel: [w223] -> w181
          tunnel: w180 -> [w222]
          tunnel: w167 -> [_]
          tunnel: w166 -> [_]
          tunnel: w165 -> [_]
          tunnel: w164 -> [_]
          frame #0 {
            n76 = call <vilib>:"Wait at Rendezvous.vi"("error in (no error)"=w224, "ms timeout (-1)"=20000, "rendezvous"=w222) -> ("error out"=w223:errorcluster)  [unwired: 2 in, 2 out]
          }
        }
        n77 = while {
          shift-right: [w257] -> w159
          shift-left: w210 -> [w255]
          tunnel: w166 -> [w252]
          tunnel: w167 -> [w249]
          tunnel: [w230] -> w179
          tunnel: [w246] -> w177
          tunnel: w165 -> [w245]
          tunnel: [w243] -> w173
          tunnel: w164 -> [w240]
          tunnel: [w228] -> w170
          shift-right: [w248] -> w178
          shift-left: w216 -> [w250]
          shift-right: [w247] -> w176
          shift-left: w217 -> [w251]
          shift-right: [w241] -> w172
          shift-left: w214 -> [w244]
          shift-right: [w237] -> w169
          shift-left: w213 -> [w238]
          tunnel: w181 -> [w256]
          tunnel: [w229] -> w161
          tunnel: [w225] -> w183
          stop <- w260 stop-if-true
          # "Run Loop"
          n78 = call-dynamic "Read Temperature DBL.vi"("error in"=w256, "IRead Temperature in"=w255) -> ("error out"=w229:errorcluster, "Time Stamp"=→"Time Stamp t":timestamp, "Temperature"=w236:dbl, "IRead Temperature out"=w257:refnum<class "IRead Temperature.lvclass">)  [unwired: 6 in]
          "Temperature" <- w236
          n79 = call-dynamic "Read Pressure DBL.vi"("error in"=w249, "IRead Pressure in"=w250) -> ("error out"=w230:errorcluster, "Time Stamp"=→"Time Stamp p":timestamp, "Pressure"=w235:dbl, "IRead Pressure out"=w248:refnum<class "IRead Pressure.lvclass">)  [unwired: 6 in]
          "Pressure" <- w235
          n80 = call-dynamic "Read Dew Point DBL.vi"("error in"=w252, "IRead Dew Point in"=w251) -> ("error out"=w246:errorcluster, "Time Stamp"=→"Time Stamp d":timestamp, "Dew Point"=w234:dbl, "IRead Dew Point out"=w247:refnum<class "IRead Dew Point.lvclass">)  [unwired: 6 in]
          "Dew Point" <- w234
          n81 = call-dynamic "Read Humidity DBL.vi"("error in"=w245, "IRead Absolute Humidity in"=w244) -> ("error out"=w243:errorcluster, "Time Stamp"=→"Time Stamp h":timestamp, "Humidity"=w233:dbl, "IRead Absolute Humidity out"=w241:refnum<class "IRead Humidity.lvclass">)  [unwired: 6 in]
          "Absolute Humidity" <- w233
          n82 = call-dynamic "Read H2O Concentration DBL.vi"("error in"=w240, "IRead Water Concentration in"=w238) -> ("error out"=w228:errorcluster, "Time Stamp"=→"Time Stamp c":timestamp, "H2O Concentration"=w232:dbl, "IRead Water Concentration out"=w237:refnum<class "IRead H2O Concentration.lvclass">)  [unwired: 6 in]
          "H2O Concentration" <- w232
          n83 = Wait Until Next ms Multiple(millisecond multiple=u32 100) -> ()  [unwired: 1 out]
          n84 = Bundle("Temperature"=w236, "Pressure"=w235, "Dew Point"=w234, "Humidity"=w233, "H2O Concentration"=w232) -> (→"Main Supply":T6)  [unwired: 1 in]
          n85 = Unbundle By Name(w228) -> ("status"=w258:bool)
          n86 = call "Read Stop Module Loop.vi"("Module Ident"="MainSupply" ("name (unnamed)")) -> ("error out"=w225:errorcluster, "Stop"=w226:bool)  [unwired: 8 in, 1 out]
          n87 = Or(x=w258, y=w226) -> (x .or. y?=w260:bool)
        }
        n88 = call "To IRunnable.vi"("error in"=w161, "LabVIEW Object"=w159) -> ("error out"=w162:errorcluster, "IRunnable"=w163:refnum<class "IRunnable.lvclass">)  [unwired: 8 in]
        n89 = call "Stop IRunable.vi"("error in"=w173, "IRunnable Object"=w172) -> ("error out"=w171:errorcluster)  [unwired: 8 in, 1 out]
        n90 = call "Stop IRunable.vi"("error in"=w179, "IRunnable Object"=w178) -> ("error out"=w174:errorcluster)  [unwired: 8 in, 1 out]
        n91 = call "Stop IRunable.vi"("error in"=w177, "IRunnable Object"=w176) -> ("error out"=w175:errorcluster)  [unwired: 8 in, 1 out]
        n92 = call "Stop IRunable.vi"("error in"=w170, "IRunnable Object"=w169) -> ("error out"=w168:errorcluster)  [unwired: 8 in, 1 out]
        n93 = call-dynamic "Stop.vi"("error in"=w162, "IRunnable in"=w163) -> ("error out"=w160:errorcluster)  [unwired: 8 in, 1 out]
        n94 = Merge Errors(w160, w174, w175, w171, w168, w183) -> (w219:errorcluster)
      }
    }
  }
  n95 = while "UI Loop" {
    tunnel: [w265] -> w14
    tunnel: w24 -> [w264]
    tunnel: [w263] -> w21
    stop <- w267 stop-if-true
    # "UI Loop"
    n96 = event shown="[2] <Close UI Loop>: User Event" {
      selector: w264 -> [_ _ _ _ _]
      dyn-events: [_ _ _ _ _] -> w263
      timeout: 500 -> [_ _ _ _ _]
      tunnel: [_ w278 _ w289 w296] -> w265
      tunnel: [_ FALSE TRUE _ _] -> w266
      event Timeout {
        w268 = enum16{"Get", "Set Temp", "Set Fan"}."Get" ("Action")
        n97 = event-data() -> ()  [unwired: 1 in, 3 out]
        n98 = call "Stack1 (FGV).vi"("Action"=w268) -> ("Stack out"=→"Stack1":T1)  [unwired: 10 in]
        n99 = call "Stack2 (FGV).vi"("Action"=w268) -> ("Stack out"=→"Stack2":T1)  [unwired: 10 in]
      }
      event "Shutdown Button": Value Change {
        w275 = "StacksTemperatureControl"
        w279 = "MainSupply"
        n100 = event-data() -> ()  [unwired: 1 in, 6 out]
        n101 = call "Write Stop Module Loop.vi"("Stop"=TRUE, "Module Ident"=w279) -> ("error out"=w281:errorcluster)  [unwired: 9 in]
        n102 = call "Enqueue State.vim"("Modul Control States"=Supply_Control_States."Shutdown" ("Supply Control States"), "Module Ident"=w279) -> ("error out"=w277:errorcluster)  [unwired: 9 in]
        n103 = call "Write Stop Module Loop.vi"("Stop"=TRUE, "Module Ident"=w275) -> ("error out"=w272:errorcluster)  [unwired: 9 in]
        n104 = call "Enqueue State.vim"("Modul Control States"=Supply_Control_States."Shutdown" ("Supply Control States"), "Module Ident"=w275) -> ("error out"=w271:errorcluster)  [unwired: 9 in]
        n105 = Merge Errors(w281, w277, w272, w271) -> (w278:errorcluster)
      }
      event User Event {
        n106 = event-data() -> ()  [unwired: 1 in, 5 out]
      }
      event "Start Button": Value Change {
        w288 = "StacksTemperatureControl"
        w292 = "MainSupply"
        n107 = event-data() -> ()  [unwired: 1 in, 6 out]
        n108 = call "Write Stop Module Loop.vi"("Stop"=FALSE, "Module Ident"=w288) -> ("error out"=w285:errorcluster)  [unwired: 9 in]
        n109 = call "Enqueue State.vim"("Modul Control States"=Supply_Control_States."Run" ("Supply Control States"), "Module Ident"=w288) -> ("error out"=w284:errorcluster)  [unwired: 9 in]
        n110 = call "Write Stop Module Loop.vi"("Stop"=FALSE, "Module Ident"=w292) -> ("error out"=w291:errorcluster)  [unwired: 9 in]
        n111 = call "Enqueue State.vim"("Modul Control States"=Supply_Control_States."Run" ("Supply Control States"), "Module Ident"=w292) -> ("error out"=w290:errorcluster)  [unwired: 9 in]
        n112 = Merge Errors(w291, w290, w285, w284) -> (w289:errorcluster)
      }
      event "Stop Button": Value Change {
        n113 = event-data() -> ()  [unwired: 1 in, 6 out]
        n114 = for {
          tunnel: Supply_Control_States."Idle" ("Supply Control States") -> [w302]
          tunnel: string[] ["MainSupply", "StacksTemperatureControl"] -> [w301] mode=indexing
          tunnel: [w298] -> w296
          n115 = call "Write Stop Module Loop.vi"("Stop"=TRUE, "Module Ident"=w301) -> ("error out"=w300:errorcluster)  [unwired: 9 in]
          n116 = call "Enqueue State.vim"("Modul Control States"=w302, "Module Ident"=w301) -> ("error out"=w299:errorcluster)  [unwired: 9 in]
          n117 = Merge Errors(w300, w299) -> (w298:errorcluster)
        }
      }
    }
    n118 = Or(x=w265, y=w266) -> (x .or. y?=w267:bool)
  }
  n119 = register-events(error in=w17, w15) -> (reference out=w38:refnum<event-registration>, error out=w36:errorcluster)  [unwired: 1 in]
  n120 = while "Alarming Loop" {
    shift-right: [w305] -> w18
    shift-left: w36 -> [w308]
    tunnel: w38 -> [w310]
    tunnel: [w309] -> w39
    stop <- w306 stop-if-true
    n121 = event shown="[1] Timeout" {
      selector: w310 -> [_ _]
      dyn-events: [_ _] -> w309
      timeout: 1000 -> [_ _]
      tunnel: w308 -> [w313 w314]
      tunnel: [w313 w314] -> w305
      tunnel: [_ w315] -> w307
      event User Event {
        n122 = event-data() -> ("Identifier"=→"Identifier":string, "Alarming Level"=→"Alarming Level":T5)  [unwired: 1 in, 4 out]
      }
      event Timeout {
        n123 = event-data() -> ()  [unwired: 1 in, 3 out]
        n124 = local read "Shutdown Button"() -> (w315:bool)
      }
    }
    n125 = Or(x=w305, y=w307) -> (x .or. y?=w306:bool)
  }
  n126 = Unregister For Events(event registration refnum=w39) -> ()  [unwired: 1 in, 1 out]
  n127 = Unregister For Events(event registration refnum=w21) -> ()  [unwired: 1 in, 1 out]
  n128 = Merge Errors(w18, w50, w20) -> (w25:errorcluster)
  n129 = call "Instrument Manager_CleanUp.vi"("Error In"=w25) -> ("Error Out"=w3:errorcluster)  [unwired: 10 in]
  n130 = flat-sequence {
    tunnel: [w317] -> w13
    tunnel: w12 -> [w319]
    tunnel: [w316] -> _
    tunnel: w3 -> [w316]
    frame #0 {
      n131 = Generate User Event "Close UI Loop"(user event=w319, event data cluster=TRUE ("event data")) -> (error out=w320:errorcluster)  [unwired: 2 in, 1 out]
      n132 = Merge Errors(w316, w320) -> (w317:errorcluster)
    }
  }
  n133 = Merge Errors(w13, w14) -> (w8:errorcluster)
  n134 = flat-sequence {
    tunnel: w8 -> [w322]
    tunnel: [w324] -> w7
    frame #0 {
      w333 = "StacksTemperatureControl"
      w330 = "MainSupply"
      n135 = Obtain Queue(name (unnamed)=w330, element data type=Supply_Control_States."Idle" ("Supply Control States")) -> (queue out=w341:refnum<queue>, error out=w342:errorcluster)  [unwired: 3 in, 1 out]
      n136 = call "Read Stop Module Loop.vi"("Module Ident"=w330) -> ("error out"=w329:errorcluster, "notifier out"=w326:refnum<notifier>)  [unwired: 8 in, 1 out]
      n137 = Release Notifier(notifier=w326, force destroy? (F)=TRUE, error in (no error)=w329) -> (error out=w325:errorcluster)  [unwired: 2 out]
      n138 = Release Queue(queue=w341, force destroy? (F)=TRUE, error in (no error)=w342) -> (error out=w339:errorcluster)  [unwired: 2 out]
      n139 = Merge Errors(w325, w339) -> (w321:errorcluster)
      n140 = Obtain Queue(name (unnamed)=w333, element data type=Supply_Control_States."Idle" ("Supply Control States")) -> (queue out=w337:refnum<queue>, error out=w338:errorcluster)  [unwired: 3 in, 1 out]
      n141 = call "Read Stop Module Loop.vi"("Module Ident"=w333) -> ("error out"=w332:errorcluster, "notifier out"=w331:refnum<notifier>)  [unwired: 8 in, 1 out]
      n142 = Release Queue(queue=w337, force destroy? (F)=TRUE, error in (no error)=w338) -> (error out=w343:errorcluster)  [unwired: 2 out]
      n143 = Release Notifier(notifier=w331, force destroy? (F)=TRUE, error in (no error)=w332) -> (error out=w323:errorcluster)  [unwired: 2 out]
      n144 = Merge Errors(w322, w321, w323, w343) -> (w324:errorcluster)
    }
  }
  n145 = disable-structure shown="Enabled" {
    disable-tunnel: [w345 w596] -> _
    disable-tunnel: errorcluster {"status"=FALSE, "code"=0, "source"=""} ("Error Out") -> [w344 w596]
    frame Disabled {
      n146 = Obtain Queue(name (unnamed)="StacksTemperatureControl", element data type=Supply_Control_States."Idle" ("Supply Control States"), error in (no error)=w344) -> (queue out=w346:refnum<queue>, error out=w347:errorcluster)  [unwired: 2 in, 1 out]
      n147 = while "Supply Loop" {
        shift-right: [w355] -> w345
        shift-left: w347 -> [w354]
        tunnel: w346 -> [w350]
        stop <- w351 stop-if-true
        # "Stacks Temperature Control"
        n148 = Dequeue Element(queue=w350, error in (no error)=w354) -> (element=w352:T7, error out=w353:errorcluster)  [unwired: 1 in, 2 out]
        n149 = case shown="\"Run\"" w352 {
          tunnel: [w356 w358 w524] -> w355
          tunnel: w353 -> [w356 w358 w376]
          tunnel: [_ TRUE _] -> w351
          frame "Idle", Default {
          }
          frame "Shutdown" {
          }
          frame "Run" {
            n150 = call "Get or Create Action Point.vi"("Error In"=w376, "Action Point Identifier"="Stack1.Temperature" ("Instrument Identifier")) -> ("Error Out"=w499:errorcluster, "IAction Point"=w497:refnum<class "IVirtual Instrument.lvclass">)  [unwired: 8 in]
            n151 = call "Get or Create Action Point.vi"("Error In"=w376, "Action Point Identifier"="Stack1.Fan") -> ("Error Out"=w449:errorcluster, "IAction Point"=w452:refnum<class "IVirtual Instrument.lvclass">)  [unwired: 8 in]
            n152 = call "Get or Create Action Point.vi"("Error In"=w376, "Action Point Identifier"="Stack2.Temperature" ("Virtual Instrument Identifier")) -> ("Error Out"=w496:errorcluster, "IAction Point"=w493:refnum<class "IVirtual Instrument.lvclass">)  [unwired: 8 in]
            n153 = call "Get or Create Action Point.vi"("Action Point Identifier"="Stack2.Fan") -> ("Error Out"=w438:errorcluster, "IAction Point"=w440:refnum<class "IVirtual Instrument.lvclass">)  [unwired: 9 in]
            n154 = call "Get or Create Action Point.vi"("Error In"=w376, "Action Point Identifier"="Stack3.Temperature" ("Instrument Identifier")) -> ("Error Out"=w490:errorcluster, "IAction Point"=w489:refnum<class "IVirtual Instrument.lvclass">)  [unwired: 8 in]
            n155 = call "Get or Create Action Point.vi"("Action Point Identifier"="Stack3.Fan") -> ("Error Out"=w423:errorcluster, "IAction Point"=w421:refnum<class "IVirtual Instrument.lvclass">)  [unwired: 9 in]
            n156 = call "Get or Create Action Point.vi"("Error In"=w376, "Action Point Identifier"="Stack4.Temperature" ("Virtual Instrument Identifier")) -> ("Error Out"=w485:errorcluster, "IAction Point"=w482:refnum<class "IVirtual Instrument.lvclass">)  [unwired: 8 in]
            n157 = call "Get or Create Action Point.vi"("Action Point Identifier"="Stack4.Fan") -> ("Error Out"=w410:errorcluster, "IAction Point"=w413:refnum<class "IVirtual Instrument.lvclass">)  [unwired: 9 in]
            n158 = call "Get or Create Action Point.vi"("Error In"=w376, "Action Point Identifier"="Stack5.Temperature" ("Virtual Instrument Identifier")) -> ("Error Out"=w479:errorcluster, "IAction Point"=w480:refnum<class "IVirtual Instrument.lvclass">)  [unwired: 8 in]
            n159 = call "Get or Create Action Point.vi"("Action Point Identifier"="Stack5.Fan") -> ("Error Out"=w402:errorcluster, "IAction Point"=w399:refnum<class "IVirtual Instrument.lvclass">)  [unwired: 9 in]
            n160 = call "Get or Create Action Point.vi"("Error In"=w376, "Action Point Identifier"="Stack6.Temperature" ("Virtual Instrument Identifier")) -> ("Error Out"=w465:errorcluster, "IAction Point"=w464:refnum<class "IVirtual Instrument.lvclass">)  [unwired: 8 in]
            n161 = call "Get or Create Action Point.vi"("Error In"=w376, "Action Point Identifier"="Stack6.Fan") -> ("Error Out"=w389:errorcluster, "IAction Point"=w392:refnum<class "IVirtual Instrument.lvclass">)  [unwired: 8 in]
            n162 = call-dynamic "Start.vi"("error in"=w496, "IRunnable in"=w493) -> ("error out"=w495:errorcluster, "IRunnable out"=w494:refnum<class "IVirtual Instrument.lvclass">)  [unwired: 8 in]
            n163 = call-dynamic "Start.vi"("error in"=w438, "IRunnable in"=w440) -> ("error out"=w437:errorcluster, "IRunnable out"=w439:refnum<class "IVirtual Instrument.lvclass">)  [unwired: 8 in]
            n164 = call-dynamic "Start.vi"("error in"=w490, "IRunnable in"=w489) -> ("error out"=w492:errorcluster, "IRunnable out"=w491:refnum<class "IVirtual Instrument.lvclass">)  [unwired: 8 in]
            n165 = call-dynamic "Start.vi"("error in"=w423, "IRunnable in"=w421) -> ("error out"=w424:errorcluster, "IRunnable out"=w422:refnum<class "IVirtual Instrument.lvclass">)  [unwired: 8 in]
            n166 = call-dynamic "Start.vi"("error in"=w485, "IRunnable in"=w482) -> ("error out"=w484:errorcluster, "IRunnable out"=w483:refnum<class "IVirtual Instrument.lvclass">)  [unwired: 8 in]
            n167 = call-dynamic "Start.vi"("error in"=w410, "IRunnable in"=w413) -> ("error out"=w411:errorcluster, "IRunnable out"=w414:refnum<class "IVirtual Instrument.lvclass">)  [unwired: 8 in]
            n168 = call-dynamic "Start.vi"("error in"=w479, "IRunnable in"=w480) -> ("error out"=w478:errorcluster, "IRunnable out"=w477:refnum<class "IVirtual Instrument.lvclass">)  [unwired: 8 in]
            n169 = call-dynamic "Start.vi"("error in"=w402, "IRunnable in"=w399) -> ("error out"=w401:errorcluster, "IRunnable out"=w398:refnum<class "IVirtual Instrument.lvclass">)  [unwired: 8 in]
            n170 = call-dynamic "Start.vi"("error in"=w389, "IRunnable in"=w392) -> ("error out"=w390:errorcluster, "IRunnable out"=w393:refnum<class "IVirtual Instrument.lvclass">)  [unwired: 8 in]
            n171 = call-dynamic "Start.vi"("error in"=w499, "IRunnable in"=w497) -> ("error out"=w502:errorcluster, "IRunnable out"=w501:refnum<class "IVirtual Instrument.lvclass">)  [unwired: 8 in]
            n172 = call-dynamic "Start.vi"("error in"=w449, "IRunnable in"=w452) -> ("error out"=w451:errorcluster, "IRunnable out"=w450:refnum<class "IVirtual Instrument.lvclass">)  [unwired: 8 in]
            n173 = call-dynamic "Start.vi"("error in"=w465, "IRunnable in"=w464) -> ("error out"=w466:errorcluster, "IRunnable out"=w467:refnum<class "IVirtual Instrument.lvclass">)  [unwired: 8 in]
            n174 = To More Specific Class(target class=refnum<class "IRead Temperature.lvclass"> refnum ("IRead Temperature.lvclass"), reference=w501, error in=w502) -> (specific class reference=w504:refnum<class "IRead Temperature.lvclass">, error out=w503:errorcluster)
            n175 = To More Specific Class(target class=refnum<class "IWrite Duty Cycle.lvclass"> refnum ("IWrite Duty Cycle.lvclass"), reference=w450, error in=w451) -> (specific class reference=w447:refnum<class "IWrite Duty Cycle.lvclass">, error out=w448:errorcluster)
            n176 = To More Specific Class(target class=refnum<class "IWrite Duty Cycle.lvclass"> refnum ("IWrite Duty Cycle.lvclass"), reference=w398, error in=w401) -> (specific class reference=w395:refnum<class "IWrite Duty Cycle.lvclass">, error out=w396:errorcluster)
            n177 = To More Specific Class(target class=refnum<class "IRead Temperature.lvclass"> refnum ("IRead Temperature.lvclass"), reference=w494, error in=w495) -> (specific class reference=w520:refnum<class "IRead Temperature.lvclass">, error out=w519:errorcluster)
            n178 = To More Specific Class(target class=refnum<class "IRead Temperature.lvclass"> refnum ("IRead Temperature.lvclass"), reference=w491, error in=w492) -> (specific class reference=w521:refnum<class "IRead Temperature.lvclass">, error out=w522:errorcluster)
            n179 = To More Specific Class(target class=refnum<class "IRead Temperature.lvclass"> refnum ("IRead Temperature.lvclass"), reference=w483, error in=w484) -> (specific class reference=w513:refnum<class "IRead Temperature.lvclass">, error out=w514:errorcluster)
            n180 = To More Specific Class(target class=refnum<class "IRead Temperature.lvclass"> refnum ("IRead Temperature.lvclass"), reference=w477, error in=w478) -> (specific class reference=w509:refnum<class "IRead Temperature.lvclass">, error out=w510:errorcluster)
            n181 = To More Specific Class(target class=refnum<class "IWrite Duty Cycle.lvclass"> refnum ("IWrite Duty Cycle.lvclass"), reference=w439, error in=w437) -> (specific class reference=w436:refnum<class "IWrite Duty Cycle.lvclass">, error out=w435:errorcluster)
            n182 = To More Specific Class(target class=refnum<class "IWrite Duty Cycle.lvclass"> refnum ("IWrite Duty Cycle.lvclass"), reference=w422, error in=w424) -> (specific class reference=w419:refnum<class "IWrite Duty Cycle.lvclass">, error out=w418:errorcluster)
            n183 = To More Specific Class(target class=refnum<class "IWrite Duty Cycle.lvclass"> refnum ("IWrite Duty Cycle.lvclass"), reference=w414, error in=w411) -> (specific class reference=w408:refnum<class "IWrite Duty Cycle.lvclass">, error out=w409:errorcluster)
            n184 = To More Specific Class(target class=refnum<class "IWrite Duty Cycle.lvclass"> refnum ("IWrite Duty Cycle.lvclass"), reference=w393, error in=w390) -> (specific class reference=w387:refnum<class "IWrite Duty Cycle.lvclass">, error out=w388:errorcluster)
            n185 = To More Specific Class(target class=refnum<class "IRead Temperature.lvclass"> refnum ("IRead Temperature.lvclass"), reference=w467, error in=w466) -> (specific class reference=w461:refnum<class "IRead Temperature.lvclass">, error out=w460:errorcluster)
            n186 = while {
              shift-right: [w594] -> w527
              shift-left: w504 -> [w592]
              tunnel: w522 -> [w586]
              tunnel: w519 -> [w588]
              tunnel: w514 -> [w584]
              tunnel: w510 -> [w582]
              shift-right: [w581] -> w516
              shift-left: w520 -> [w589]
              shift-right: [w580] -> w517
              shift-left: w521 -> [w587]
              shift-right: [w579] -> w512
              shift-left: w513 -> [w585]
              shift-right: [w578] -> w506
              shift-left: w509 -> [w583]
              tunnel: w503 -> [w593]
              tunnel: [w566] -> w529
              tunnel: [w591] -> w468
              tunnel: w460 -> [w544]
              tunnel: [w577] -> w459
              tunnel: [w576] -> w458
              tunnel: [w575] -> w457
              tunnel: [w574] -> w456
              tunnel: w448 -> [w569]
              shift-right: [w568] -> w445
              shift-left: w447 -> [w571]
              tunnel: [w567] -> w446
              shift-right: [w562] -> w432
              shift-left: w436 -> [w565]
              shift-right: [w561] -> w433
              shift-left: w435 -> [w564]
              tunnel: w419 -> [w559]
              tunnel: w418 -> [w558]
              shift-right: [w556] -> _
              shift-left: TRUE -> [w538]
              tunnel: [w555] -> w416
              tunnel: w409 -> [w554]
              shift-right: [w548] -> w403
              shift-left: w408 -> [w553]
              tunnel: [w549] -> w405
              shift-right: [w532] -> w383
              shift-left: w395 -> [w541]
              tunnel: w396 -> [w547]
              tunnel: w388 -> [w542]
              tunnel: [w537] -> w375
              shift-right: [w536] -> w374
              shift-left: w387 -> [w540]
              shift-right: [w535] -> w378
              shift-left: w461 -> [w543]
              tunnel: [w534] -> w379
              tunnel: [w533] -> w384
              stop <- w530 stop-if-true
              w556 = FALSE  # reinit pids
              # "Run Loop"
              n187 = call-dynamic "Read Temperature DBL.vi"("error in"=w593, "IRead Temperature in"=w592) -> ("error out"=w566:errorcluster, "Temperature"=w572:dbl, "IRead Temperature out"=w594:refnum<class "IRead Temperature.lvclass">)  [unwired: 6 in, 1 out]
              n188 = call-dynamic "Read Temperature DBL.vi"("error in"=w586, "IRead Temperature in"=w587) -> ("error out"=w575:errorcluster, "Temperature"=w552:dbl, "IRead Temperature out"=w580:refnum<class "IRead Temperature.lvclass">)  [unwired: 6 in, 1 out]
              n189 = call-dynamic "Read Temperature DBL.vi"("error in"=w588, "IRead Temperature in"=w589) -> ("error out"=w574:errorcluster, "Temperature"=w560:dbl, "IRead Temperature out"=w581:refnum<class "IRead Temperature.lvclass">)  [unwired: 6 in, 1 out]
              n190 = call-dynamic "Read Temperature DBL.vi"("error in"=w584, "IRead Temperature in"=w585) -> ("error out"=w576:errorcluster, "Temperature"=w550:dbl, "IRead Temperature out"=w579:refnum<class "IRead Temperature.lvclass">)  [unwired: 6 in, 1 out]
              n191 = call-dynamic "Read Temperature DBL.vi"("error in"=w582, "IRead Temperature in"=w583) -> ("error out"=w577:errorcluster, "Temperature"=w545:dbl, "IRead Temperature out"=w578:refnum<class "IRead Temperature.lvclass">)  [unwired: 6 in, 1 out]
              n192 = call-dynamic "Read Temperature DBL.vi"("error in"=w544, "IRead Temperature in"=w543) -> ("error out"=w534:errorcluster, "Temperature"=w531:dbl, "IRead Temperature out"=w535:refnum<class "IRead Temperature.lvclass">)  [unwired: 6 in, 1 out]
              n193 = call "Stack PID Fan.vi"("Reinitialize"=w538, "Temperature"=w552) -> ("Output"=w557:dbl)  [unwired: 9 in]
              n194 = call "Stack PID Fan.vi"("Reinitialize"=w538, "Temperature"=w560) -> ("Output"=w563:dbl)  [unwired: 9 in]
              n195 = call "Stack PID Fan.vi"("Reinitialize"=w538, "Temperature"=w572) -> ("Output"=w570:dbl)  [unwired: 9 in]
              n196 = call "Stack PID Fan.vi"("Reinitialize"=w538, "Temperature"=w545) -> ("Output"=w546:dbl)  [unwired: 9 in]
              n197 = call "Stack PID Fan.vi"("Reinitialize"=w538, "Temperature"=w531) -> ("Output"=w539:dbl)  [unwired: 9 in]
              n198 = call "Stack PID Fan.vi"("Reinitialize"=w538, "Temperature"=w550) -> ("Output"=w551:dbl)  [unwired: 9 in]
              n199 = call-dynamic "Write Duty Cycle %.vi"("error in"=w564, "Duty Cycle"=w563, "IWrite Duty Cycle in"=w565) -> ("error out"=w561:errorcluster, "IWrite Duty Cycle out"=w562:refnum<class "IWrite Duty Cycle.lvclass">)  [unwired: 7 in]
              n200 = call-dynamic "Write Duty Cycle %.vi"("error in"=w558, "Duty Cycle"=w557, "IWrite Duty Cycle in"=w559) -> ("error out"=w555:errorcluster)  [unwired: 7 in, 1 out]
              n201 = call-dynamic "Write Duty Cycle %.vi"("error in"=w554, "Duty Cycle"=w551, "IWrite Duty Cycle in"=w553) -> ("error out"=w549:errorcluster, "IWrite Duty Cycle out"=w548:refnum<class "IWrite Duty Cycle.lvclass">)  [unwired: 7 in]
              n202 = call-dynamic "Write Duty Cycle %.vi"("error in"=w569, "Duty Cycle"=w570, "IWrite Duty Cycle in"=w571) -> ("error out"=w567:errorcluster, "IWrite Duty Cycle out"=w568:refnum<class "IWrite Duty Cycle.lvclass">)  [unwired: 7 in]
              n203 = call-dynamic "Write Duty Cycle %.vi"("error in"=w542, "Duty Cycle"=w539, "IWrite Duty Cycle in"=w540) -> ("error out"=w537:errorcluster, "IWrite Duty Cycle out"=w536:refnum<class "IWrite Duty Cycle.lvclass">)  [unwired: 7 in]
              n204 = call-dynamic "Write Duty Cycle %.vi"("error in"=w547, "Duty Cycle"=w546, "IWrite Duty Cycle in"=w541) -> ("error out"=w533:errorcluster, "IWrite Duty Cycle out"=w532:refnum<class "IWrite Duty Cycle.lvclass">)  [unwired: 7 in]
              n205 = Wait Until Next ms Multiple(millisecond multiple=u32 1000) -> ()  [unwired: 1 out]
              n206 = Bundle("Temperature"=w572, "Temperature"=w560, "Temperature"=w552, "Temperature"=w550, "Temperature"=w545, "Temperature"=w531) -> (→"Stack Temperatures":T4)  [unwired: 1 in]
              n207 = call "Read Stop Module Loop.vi"("Module Ident"="StacksTemperatureControl" ("name (unnamed)")) -> ("error out"=w591:errorcluster, "Stop"=w530:bool)  [unwired: 8 in, 1 out]
            }
            n208 = To More Specific Class(target class=refnum<class "IRunnable.lvclass"> refnum ("IRunnable.lvclass"), reference=w374, error in=w375) -> (specific class reference=w372:refnum<class "IRunnable.lvclass">, error out=w373:errorcluster)
            n209 = To More Specific Class(target class=refnum<class "IRunnable.lvclass"> refnum ("IRunnable.lvclass"), reference=w383, error in=w384) -> (specific class reference=w386:refnum<class "IRunnable.lvclass">, error out=w385:errorcluster)
            n210 = To More Specific Class(target class=refnum<class "IRunnable.lvclass"> refnum ("IRunnable.lvclass"), reference=w378, error in=w379) -> (specific class reference=w380:refnum<class "IRunnable.lvclass">, error out=w381:errorcluster)
            n211 = To More Specific Class(target class=refnum<class "IRunnable.lvclass"> refnum ("IRunnable.lvclass"), reference=w527, error in=w529) -> (specific class reference=w500:refnum<class "IRunnable.lvclass">, error out=w528:errorcluster)
            n212 = To More Specific Class(target class=refnum<class "IRunnable.lvclass"> refnum ("IRunnable.lvclass"), reference=w445, error in=w446) -> (specific class reference=w442:refnum<class "IRunnable.lvclass">, error out=w443:errorcluster)
            n213 = To More Specific Class(target class=refnum<class "IRunnable.lvclass"> refnum ("IRunnable.lvclass"), reference=w516, error in=w456) -> (specific class reference=w475:refnum<class "IRunnable.lvclass">, error out=w476:errorcluster)
            n214 = To More Specific Class(target class=refnum<class "IRunnable.lvclass"> refnum ("IRunnable.lvclass"), reference=w432, error in=w433) -> (specific class reference=w430:refnum<class "IRunnable.lvclass">, error out=w429:errorcluster)
            n215 = To More Specific Class(target class=refnum<class "IRunnable.lvclass"> refnum ("IRunnable.lvclass"), error in=w416) -> (specific class reference=w428:refnum<class "IRunnable.lvclass">, error out=w427:errorcluster)  [unwired: 1 in]
            n216 = To More Specific Class(target class=refnum<class "IRunnable.lvclass"> refnum ("IRunnable.lvclass"), reference=w512, error in=w458) -> (specific class reference=w471:refnum<class "IRunnable.lvclass">, error out=w472:errorcluster)
            n217 = To More Specific Class(target class=refnum<class "IRunnable.lvclass"> refnum ("IRunnable.lvclass"), reference=w403, error in=w405) -> (specific class reference=w407:refnum<class "IRunnable.lvclass">, error out=w406:errorcluster)
            n218 = To More Specific Class(target class=refnum<class "IRunnable.lvclass"> refnum ("IRunnable.lvclass"), reference=w506, error in=w459) -> (specific class reference=w469:refnum<class "IRunnable.lvclass">, error out=w470:errorcluster)
            n219 = To More Specific Class(target class=refnum<class "IRunnable.lvclass"> refnum ("IRunnable.lvclass"), reference=w517, error in=w457) -> (specific class reference=w473:refnum<class "IRunnable.lvclass">, error out=w474:errorcluster)
            n220 = call-dynamic "Stop.vi"("error in"=w385, "IRunnable in"=w386) -> ("error out"=w368:errorcluster)  [unwired: 8 in, 1 out]
            n221 = call-dynamic "Stop.vi"("error in"=w381, "IRunnable in"=w380) -> ("error out"=w369:errorcluster)  [unwired: 8 in, 1 out]
            n222 = call-dynamic "Stop.vi"("error in"=w528, "IRunnable in"=w500) -> ("error out"=w359:errorcluster)  [unwired: 8 in, 1 out]
            n223 = call-dynamic "Stop.vi"("error in"=w443, "IRunnable in"=w442) -> ("error out"=w360:errorcluster)  [unwired: 8 in, 1 out]
            n224 = call-dynamic "Stop.vi"("error in"=w476, "IRunnable in"=w475) -> ("error out"=w361:errorcluster)  [unwired: 8 in, 1 out]
            n225 = call-dynamic "Stop.vi"("error in"=w429, "IRunnable in"=w430) -> ("error out"=w362:errorcluster)  [unwired: 8 in, 1 out]
            n226 = call-dynamic "Stop.vi"("error in"=w474, "IRunnable in"=w473) -> ("error out"=w363:errorcluster)  [unwired: 8 in, 1 out]
            n227 = call-dynamic "Stop.vi"("error in"=w427, "IRunnable in"=w428) -> ("error out"=w364:errorcluster)  [unwired: 8 in, 1 out]
            n228 = call-dynamic "Stop.vi"("error in"=w472, "IRunnable in"=w471) -> ("error out"=w365:errorcluster)  [unwired: 8 in, 1 out]
            n229 = call-dynamic "Stop.vi"("error in"=w406, "IRunnable in"=w407) -> ("error out"=w366:errorcluster)  [unwired: 8 in, 1 out]
            n230 = call-dynamic "Stop.vi"("error in"=w470, "IRunnable in"=w469) -> ("error out"=w367:errorcluster)  [unwired: 8 in, 1 out]
            n231 = call-dynamic "Stop.vi"("error in"=w373, "IRunnable in"=w372) -> ("error out"=w370:errorcluster)  [unwired: 8 in, 1 out]
            n232 = Merge Errors(w359, w360, w361, w362, w363, w364, w365, w366, w367, w368, w369, w370, w468) -> (w524:errorcluster)
          }
        }
      }
    }
    frame Enabled {
    }
  }
  "Error Out" <- w7
